vi "Multi_Run_Prog.vi"(0 "Command filename":path, 1 "Setup mode":T9(ring)) -> ()   [LabVIEW 2011]
uses:
  Anemometry Sub Vis/Globals/Trav_pos_global.vi
  Anemometry Sub Vis/Globals/Meas_global.vi
  ADAM Client/Sub VIs/ADAM Controls/Traverse_Level_State.ctl
  Anemometry Sub Vis/Gen Trav/Route mapping/Route_mapping_global.vi
  Anemometry Sub Vis/Globals/Preference_global.vi
  ADAM Client/Sub VIs/ADAM Controls/Client_Source_Status.ctl
  Anemometry Sub Vis/Controls/Multi_Run_Case.ctl
  Anemometry Sub Vis/Controls/User_Specific_mode.ctl
  ADAM Client/Sub VIs/ADAM Controls/Update_scan_value.ctl
  Anemometry Sub Vis/Controls/Multi_run_mode.ctl
  Anemometry Sub Vis/Gen Trav/Multi_Run_Status.ctl
  Anemometry Sub Vis/Globals/Extra_Commands_Global.vi
  Anemometry Sub Vis/Globals/LDA_meas_global_1.vi
  Anemometry Sub Vis/Globals/LDA_meas_global_2.vi
  ADAM Client/Sub VIs/ADAM Controls/Tunnel_speed_mode.ctl
  ADAM Client/Sub VIs/ADAM Controls/Remember_value_mode.ctl
  Anemometry Sub Vis/Controls/Overhead.ctl
  Anemometry Sub Vis/Controls/Post_Process.ctl
  Anemometry Sub Vis/Gen Trav/Spacing.ctl
  Anemometry Sub Vis/Gen Trav/Traverse_cluster.ctl
  Anemometry Sub Vis/Gen Trav/Trav_mode.ctl
  Anemometry Sub Vis/File/Setup_Filetype.ctl
  Anemometry Sub Vis/Controls/Tunnel_Coordinates.ctl
  Anemometry Sub Vis/Gen Trav/Route mapping/Route_Display_Mode.ctl
panel:
  out "Last Row Run":i32
  in  "Stop after Repeats":bool
  in  "Jump Bad Positions":bool
  in  "Work in Tunnel Coordinates?":T1
  out "Current Overhead Factor":dbl format="%.3f"
  out "Estimated Completion time":string
  out "Max Tunnel Speed":dbl format="%.2f"
  out "Pause message":string
  in  "Pause":bool
  out "Non Starter":bool
  out "No of Rows":i32
  out "Status":T2
  in  "Synchronization Start No":i32=1 min=1 max=100
  out "Multi Run Case":T3
  out "Simulate/Run":T4
  in  "Display Mode":T5=enum."Display View on Crash"
  in  "stop":bool
  out "Currently on Row":i32
  in  "Table":T6[](array[typedef]) {"Row Duration (mins)" format="%#.1f"; "Row No" min=0; "Trace Gas Concentration (%)" min=0.0 format="%#.2f"; "Emission Rate (l/min)" format="%#.2f"; "Tunnel Speed" format="%#.2f"; "Start X" format="%#.2f"; "Start Y" format="%#.2f"; "Start Z" format="%#.2f"; "End X" format="%#.2f"; "End Y" format="%#.2f"; "End Z" format="%#.2f"; "Averaging time (min)" min=0.0 format="%#.2f"}
  # "X           Y            Z"
  # "Start"
  # "End"
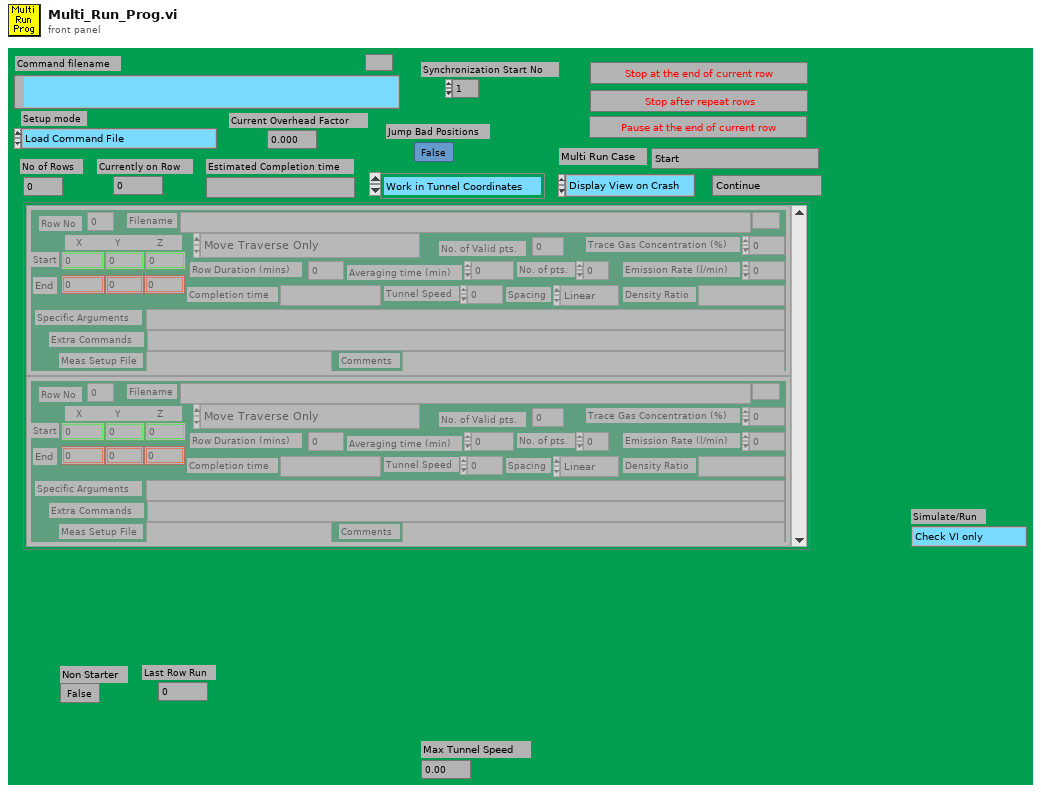
[diagram p1: front panel]
types:
  T1 = typedef "Tunnel_Coordinates.ctl" = enum16{"Work in Tunnel Coordinates", "Work in Model Coordinates"}
  T2 = typedef "Multi_Run_Status.ctl" = enum16{"Continue", "Jump to Next Point", "Jump to Next Row", "Jump To Fall Back", "Terminate Run"}
  T3 = typedef "Multi_Run_Case.ctl" = enum16{"Start", "Load Setup From File", "Has file been edited in Excel?", "Check Max Tunnel Speed", "Pre Check Row", "Check Rows", "Remove blank end rows", "Do results files already exist?", "FFID Bkgnd Measurements?", "First Save Setup file", "Setup Route checking", "Initialise Measurement Prog", "Input Current Position", "Experimental setup control", "Check source flowrates", "Setup for running mode", "Skip Blank Rows", "Which row to execute next", "Evaluate IF Statement", "Perform Measurement Setup", "Set Measurement Conditions", "Execute Row", "Calculate Row TIme", "Update time estimate", "Pause Multi Run Program", "Do Another Row?", "Find Next Fall Back Row", "Shut down source etc", "Email results to users", "Save run efficiency", "Remove Skipped Commands", "Show jumped positions", "Save Setup to File", "End"}
  T4 = typedef "User_Specific_mode.ctl" = enum16{"Check VI only", "Run VI"}
  T5 = typedef "Route_Display_Mode.ctl" = enum16{"Display View Always", "Display View on Crash"}
  T6 = typedef "Traverse_cluster.ctl" = cluster{"Start X":dbl, "Start Y":dbl, "Start Z":dbl, "End X":dbl, "End Y":dbl, "End Z":dbl, "No. of pts.":i32, "Spacing":T7, "Filename":path, "Tunnel Speed":dbl, "Averaging time (min)":dbl, "Extra Commands":string, "Specific Arguments":string, "Emission Rate (l/min)":dbl, "Trace Gas Concentration (%)":dbl, "Density Ratio":string, "Comments":string, "Row No":i32, "Row Type Selector":T8, "Completion time":string, "Row Duration (mins)":dbl, "No. of Valid pts.":i32, "Meas Setup File":string}
  T7 = typedef "Spacing.ctl" = enum16{"Linear", "Log", "Gauss", "Specified", "N/A"}
  T8 = typedef "Multi_run_mode.ctl" = enum16{"Move Traverse Only", "Set Tunnel Speed Only", "Set Source Only", "Set Measurement Conditions", "Single Measurement", "Vertical Profile", "Lateral Profile", "Longitudinal Profile", "Explore Volume", "Multi-Axis Profile", "Auto Calibrate", "Meas Fast FID Bkgnd", "Check Beam Power", "Scanning Valve Measurement", "Run VI Named:", "Set ADAM Ch", "Wait (minutes)", "Send Message", "Synchronize With:", "Fall Back to this Row", "Turn Off Row Repeating", "Blank Row"}
  T9 = enum16{"Load Command File", "Save Command File", "Check Multi Run Prog", "Check Multi Run Prog With Live Moves", "Run Multi Run Prog"}
  T10 = typedef "Post_Process.ctl" = enum16{"Take New Data", "Post Process Raw Data File"}
  T11 = typedef "Traverse_Level_State.ctl" = enum16{"Running", "Complete"}
  T12 = enum32{"existing file", "new file", "new or existing file", "existing dir", "new dir", "new or existing dir", "existing file (use LLBs)", "new file (use LLBs)", "new or existing file (use LLBs)", "new or existing file or directory (use LLBs)"}
  T13 = typedef "Tunnel_speed_mode.ctl" = enum16{"Set Speed", "Set Speed then wait", "Is tunnel speed allowable?"}
  T14 = enum16{"All Channel Names", "Valid Channel Names"}
  T15 = typedef "Overhead.ctl" = enum16{"Update total times", "Read Current Overhead", "Re Scale totals to 3 hrs", "Initialise totals to 3hr"}
  T16 = typedef "Remember_value_mode.ctl" = enum16{"Read only", "Read and Write"}
  T17 = typedef "Trav_mode.ctl" = enum16{"Move traverse", "Read traverse position", "Teach Position"}
  T18 = typedef "Client_Source_Status.ctl" = enum16{"Not Using", "Using", "Must Have"}
  T19 = typedef "Update_scan_value.ctl" = cluster{"Channel Name":string, "New Value":dbl}
  T20 = typedef "Setup_Filetype.ctl" = enum16{"Measurement Setups", "Calibration Setups", "General", "Results File Plotter Setups", "Speed Calib Tweaks"}
  T21 = typedef "Status_Cluster.ctl" = cluster{"Status":T2, "Error Type":string, "Error Description":string}
  T22 = typedef "BSA_info_Cluster.ctl" = cluster{"GPIB Address":string, "No of Check Bytes":i32, "Extra Info":string, "COLOUR":u32, "Wavelength (nm)":dbl}
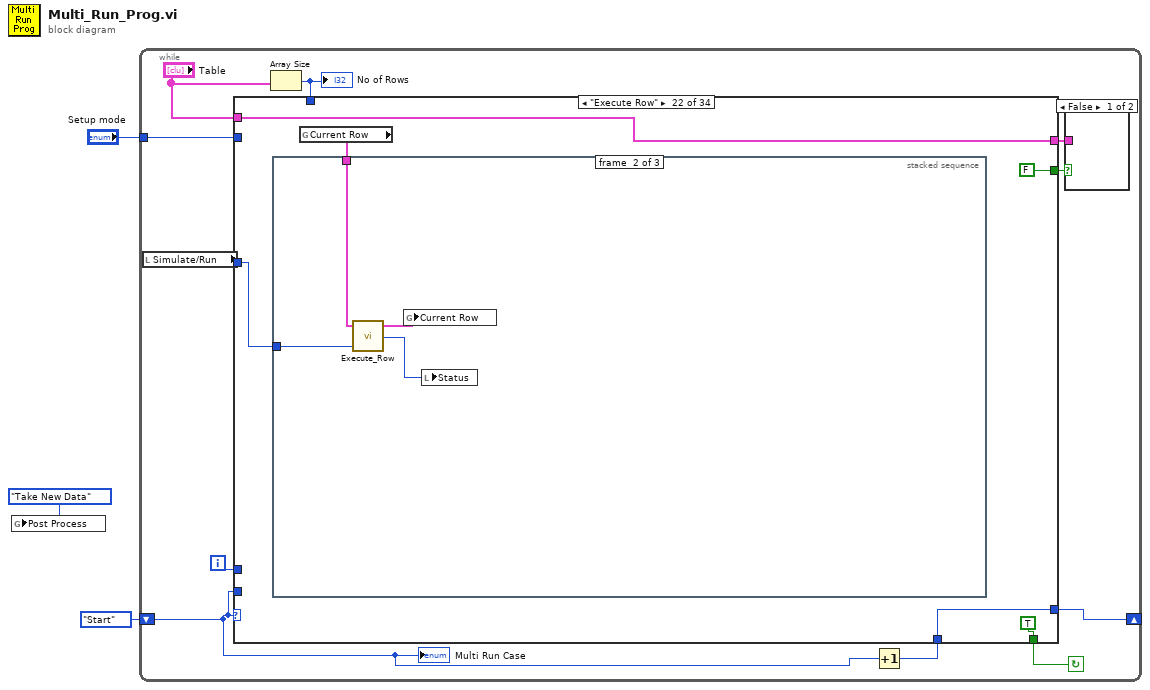
[diagram p0: block diagram]
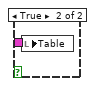
[diagram p2: hidden frame]
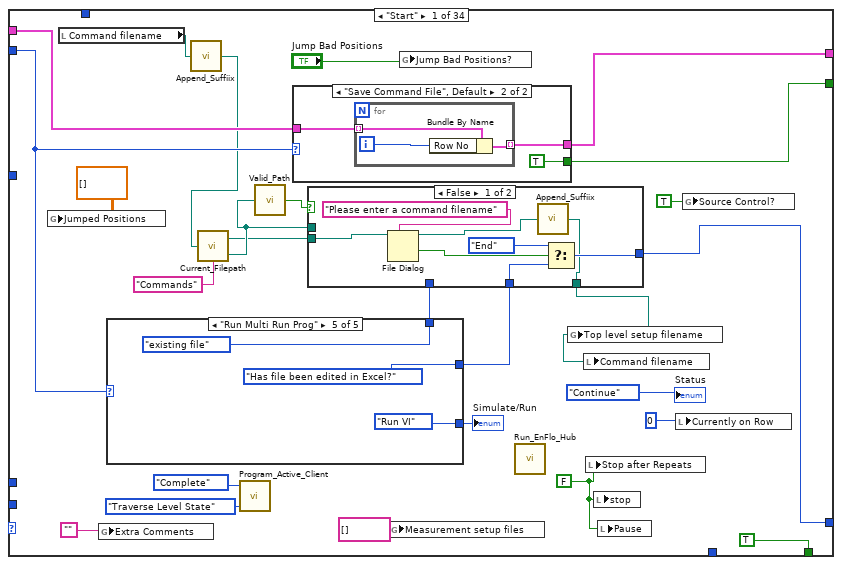
[diagram p3: hidden frame]
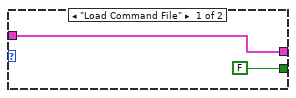
[diagram p4: hidden frame]
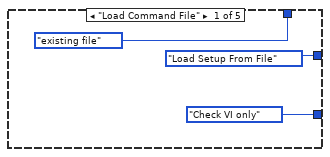
[diagram p6: hidden frame]
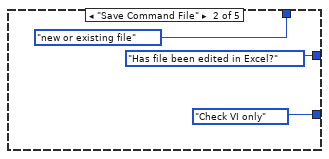
[diagram p7: hidden frame]
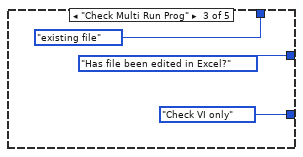
[diagram p8: hidden frame]
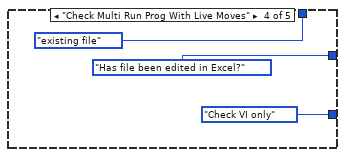
[diagram p9: hidden frame]
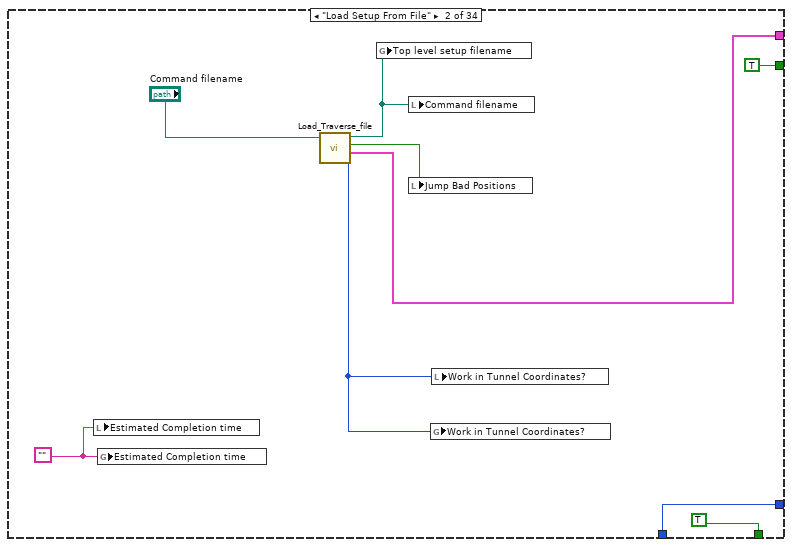
[diagram p10: hidden frame]
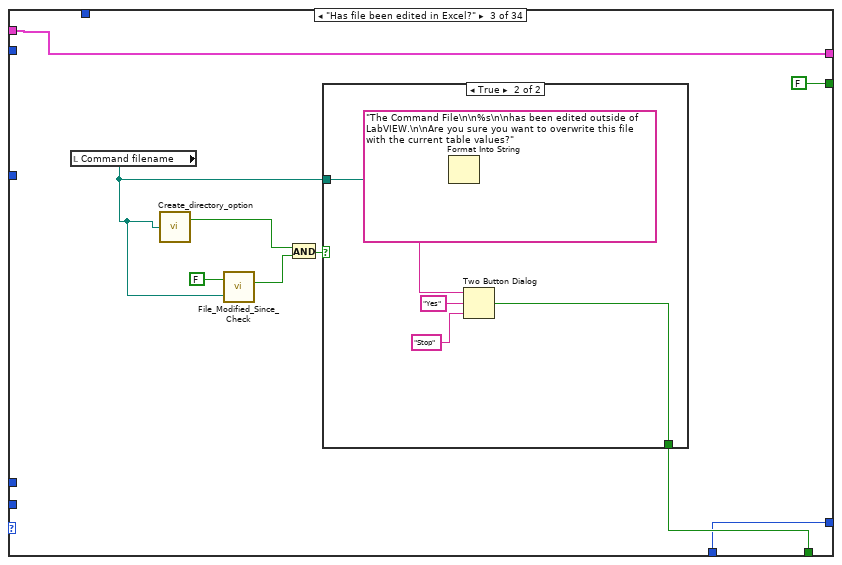
[diagram p11: hidden frame]
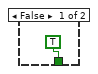
[diagram p12: hidden frame]
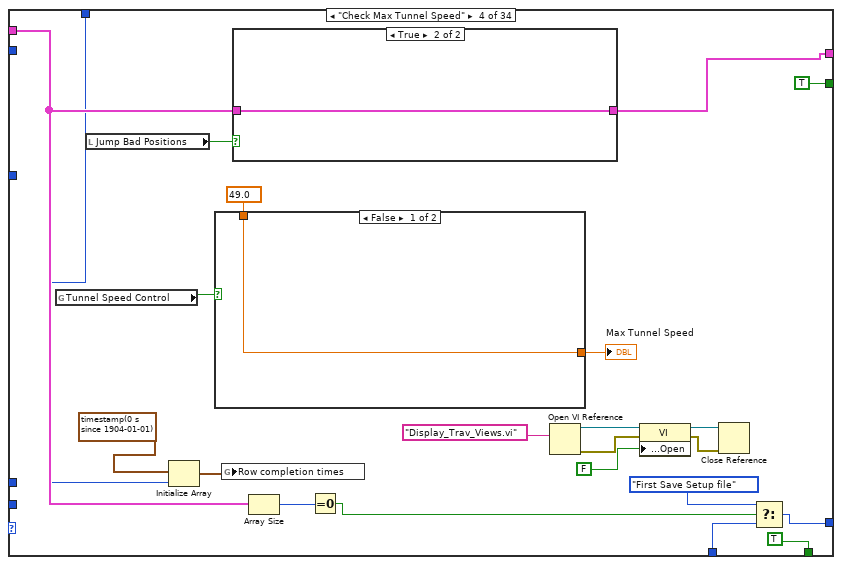
[diagram p13: hidden frame]
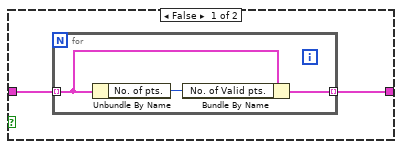
[diagram p14: hidden frame]
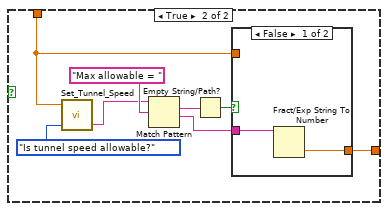
[diagram p15: hidden frame]
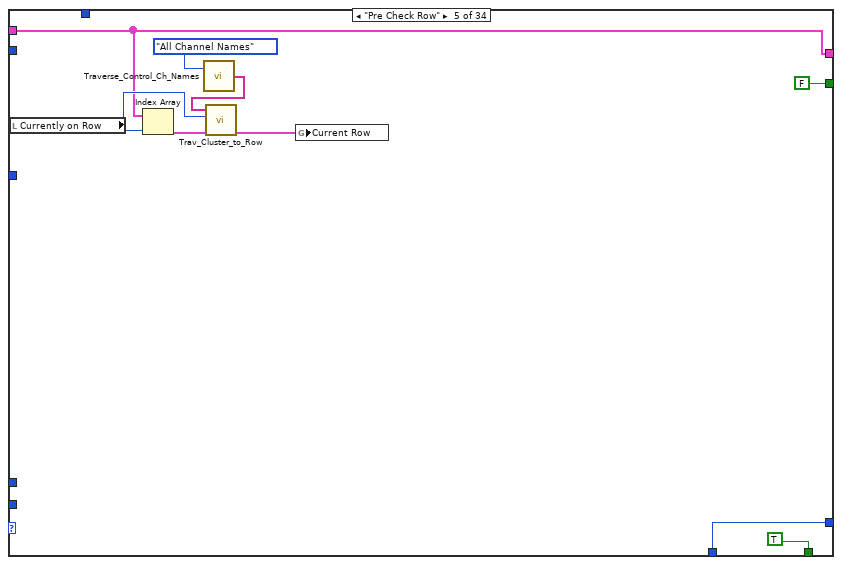
[diagram p17: hidden frame]
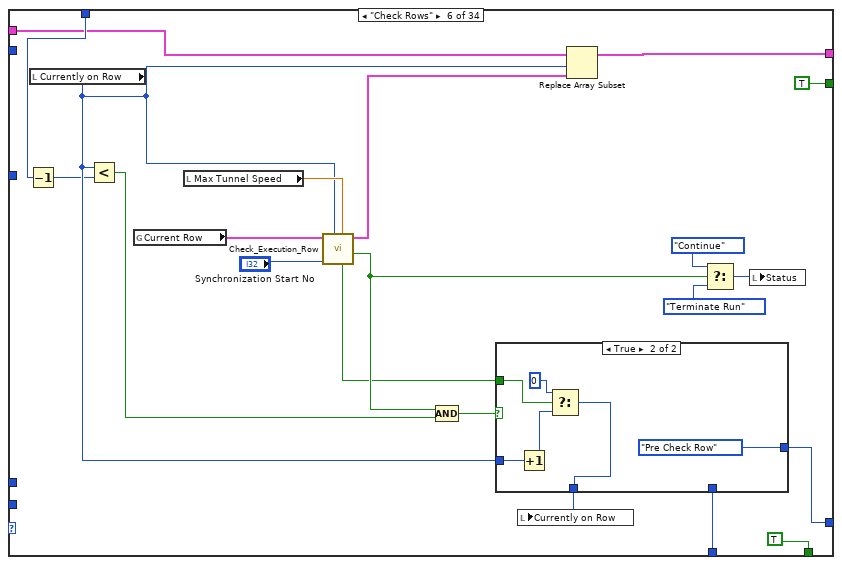
[diagram p18: hidden frame]
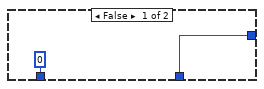
[diagram p19: hidden frame]
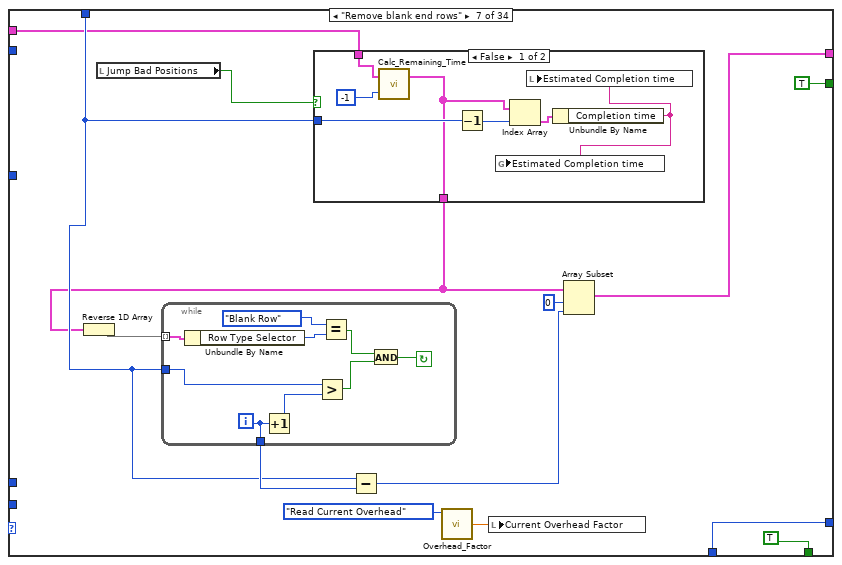
[diagram p20: hidden frame]
diagram:
  n1 = global write "Meas_global.vi" "Post Process"(Post_Process."Take New Data" ("Post Process")) -> ()
  n2 = while {
    shift-left: Multi_Run_Case."Start" ("Multi Run Case") -> [w10]
    shift-right: [w6] -> _
    tunnel: "Setup mode" -> [w13]
    i -> [w11]
    stop <- w14 continue-if-true
    n3 = local read "Simulate/Run"() -> (w7:T4)
    n4 = Array Size(array="Table") -> (size(s)=w5:i32)
    "No of Rows" <- w5
    n5 = Increment(x=w10) -> (x+1=w12:T3)
    n6 = case shown="\"Execute Row\"" w10 {
      tunnel: [TRUE TRUE w87 TRUE TRUE TRUE TRUE TRUE TRUE TRUE TRUE ("Continue?") TRUE ("Continue?") TRUE TRUE TRUE w508 TRUE ("Continue?") TRUE ("Continue?") TRUE TRUE ("Continue?") TRUE TRUE TRUE TRUE TRUE TRUE TRUE TRUE TRUE TRUE TRUE TRUE TRUE FALSE] -> w14
      tunnel: w13 -> [w26 _ _ _ _ _ _ _ _ w395 _ _ _ _ _ _ _ _ _ _ _ _ _ _ _ _ _ _ _ _ _ _ w1222 _]
      tunnel: "Table" -> [w39 _ w84 w114 w142 w154 w179 w210 w368 w397 w416 w444 w457 w485 w495 w511 w563 w607 w723 w774 w786 w877 w913 w945 w986 w1028 w1063 w1093 w1122 w1167 w1172 w1181 w1243 w1306]
      tunnel: w7 -> [_ _ _ _ _ _ _ w209 _ _ _ _ _ w489 w494 w510 _ w605 w720 w771 w784 w876 w911 w942 _ w1037 _ w1084 _ _ _ _ w1233 _]
      tunnel: w10 -> [_ _ _ _ _ _ _ _ _ _ _ _ _ _ _ _ _ _ _ _ _ _ _ _ _ _ _ _ _ _ _ _ _ _]
      tunnel: w12 -> [_ w80 w86 w112 w146 w156 w190 w214 w363 w394 w420 w441 w458 w484 w500 w513 w565 w603 w728 w775 w793 w874 w903 w947 w989 _ _ w1077 w1124 w1169 w1175 w1189 w1241 w1305]
      tunnel: w11 -> [_ _ _ _ _ _ _ _ _ _ _ _ _ _ _ _ _ _ _ _ _ _ _ _ w987 _ _ _ _ _ _ _ _ _]
      tunnel: [w37 w80 w86 w111 w146 w155 w190 w214 w363 w390 w420 w440 w458 w484 w497 w513 w565 w604 w727 w775 w794 w874 w903 w947 w990 w1038 w1060 w1088 w1124 w1169 w1175 w1189 w1241 w1305] -> w6
      tunnel: [w25 TRUE FALSE ("Rows Added ?") TRUE ("Rows Added ?") FALSE TRUE TRUE FALSE FALSE TRUE FALSE FALSE FALSE FALSE FALSE TRUE FALSE ("Rows Added ?") FALSE ("Rows Added ?") FALSE FALSE ("Rows Added ?") FALSE FALSE FALSE TRUE ("Rows Added ?") FALSE FALSE FALSE FALSE FALSE FALSE TRUE TRUE TRUE FALSE] -> w8
      tunnel: w5 -> [_ _ _ w106 _ w160 w181 _ _ _ _ _ _ _ _ _ w566 w606 _ _ _ _ _ w941 _ w1023 _ _ _ _ _ _ _ _]
      tunnel: [w38 w81 w84 w116 w142 w163 w185 w210 w368 w398 w416 w444 w457 w485 w495 w509 w563 w608 w723 w774 w786 w877 w913 w944 w986 w1028 w1063 w1093 w1122 w1167 w1171 w1181 w1242 w1306] -> w4
      frame "Start" {
        w23 = FALSE ("Measurment setup Found?")
        n7 = global write "Trav_pos_global.vi" "Jumped Positions"(dbl[][] [] ("Jumped Positions")) -> ()
        n8 = local read "Command filename"() -> (w29:path)
        n9 = global write "Meas_global.vi" "Extra Comments"("") -> ()
        n10 = case shown="\"Run Multi Run Prog\"" w26 {
          tunnel: [User_Specific_mode."Check VI only" ("Simulate/Run") User_Specific_mode."Check VI only" ("Simulate/Run") User_Specific_mode."Check VI only" ("Simulate/Run") User_Specific_mode."Check VI only" ("Simulate/Run") User_Specific_mode."Run VI" ("Simulate/Run")] -> w40
          tunnel: [Multi_Run_Case."Load Setup From File" ("Multi Run Case") Multi_Run_Case."Has file been edited in Excel?" ("Multi Run Case") Multi_Run_Case."Has file been edited in Excel?" ("Multi Run Case") Multi_Run_Case."Has file been edited in Excel?" ("Multi Run Case") Multi_Run_Case."Has file been edited in Excel?" ("Multi Run Case")] -> w36
          tunnel: [T12."existing file" ("select mode (2)") T12."new or existing file" ("select mode (2)") T12."existing file" ("select mode (2)") T12."existing file" ("select mode (2)") T12."existing file" ("select mode (2)")] -> w24
          frame "Load Command File" {
          }
          frame "Save Command File" {
          }
          frame "Check Multi Run Prog" {
          }
          frame "Check Multi Run Prog With Live Moves" {
          }
          frame "Run Multi Run Prog" {
          }
        }
        "Simulate/Run" <- w40
        n11 = call "Append_Suffiix.vi"("Results file"=w29) -> ("appended path"=w18:path)
        n12 = call "Current_Filepath.vi"("Filename in"=w18, "Data Type"="Commands") -> ("Filename Out"=w17:path, "Directory"=w16:path)
        n13 = call "Program_Active_Client.vi"("Mode"=enum16{"Program Active", "Traverse Level State"}."Traverse Level State", "Traverse level State"=Traverse_Level_State."Complete") -> ()  [unwired: 1 in, 3 out]
        n14 = call "Valid_Path.vi"("Filename"=w17) -> ("Valid Path?"=w27:bool)
        n15 = case shown="\"Save Command File\", Default" w26 {
          tunnel: w39 -> [w43 w46]
          tunnel: [w43 w45] -> w38
          tunnel: [FALSE TRUE] -> w25
          frame "Load Command File" {
          }
          frame "Save Command File", Default {
            n16 = for {
              tunnel: w46 -> [w49] mode=indexing
              tunnel: [w48] -> w45 mode=indexing
              i -> [w47]
              n17 = Bundle By Name(cluster=w49, "Row No"=w47) -> (w48:T6)
            }
          }
        }
        n18 = case shown="False" w27 {
          tunnel: [w55 w59] -> w37
          tunnel: w36 -> [w56 w59]
          tunnel: w17 -> [_ w58]
          tunnel: [w54 w58] -> w28
          tunnel: w24 -> [_ _]
          tunnel: w16 -> [w50 _]
          frame False {
            n19 = File Dialog(7:"Please enter a command filename" ("prompt"), 11:w50) -> (1:w52:bool, 3:w53:path)  [unwired: 1 in, 6 out]
            n20 = call "Append_Suffiix.vi"("Results file"=w53) -> ("appended path"=w54:path)
            n21 = Select(t=Multi_Run_Case."End" ("Multi Run Case"), s=w52, f=w56) -> (s? t:f=w55:T3)
          }
          frame True {
          }
        }
        n22 = global write "Trav_pos_global.vi" "Measurement setup files"(string[] [] ("Measurement setup files")) -> ()
        n23 = global write "Trav_pos_global.vi" "Jump Bad Positions?"("Jump Bad Positions") -> ()
        n24 = call "Run_EnFlo_Hub.vi"() -> ()  [unwired: 8 out]
        n25 = global write "Trav_pos_global.vi" "Top level setup filename"(w28) -> ()
        n26 = local write "Command filename"(w28) -> ()
        n27 = local write "Stop after Repeats"(w23) -> ()
        n28 = local write "stop"(w23) -> ()
        n29 = local write "Pause"(w23) -> ()
        n30 = local write "Currently on Row"(0 ("Currently on Row")) -> ()
        n31 = global write "Trav_pos_global.vi" "Source Control?"(TRUE ("Source Control?")) -> ()
        "Status" <- Multi_Run_Status."Continue" ("Status")
      }
      frame "Load Setup From File" {
        w76 = ""
        n32 = local write "Estimated Completion time"(w76) -> ()
        n33 = global write "Trav_pos_global.vi" "Estimated Completion time"(w76) -> ()
        n34 = call "Load_Traverse_file.vi"("Setup filename"="Command filename") -> ("Setup filename Out"=w78:path, "Jump Bad Positions"=w75:bool, "Table"=w81:T6[], "Work in Tunnel Coordinates?"=w77:T1)  [unwired: 2 out]
        n35 = global write "Trav_pos_global.vi" "Top level setup filename"(w78) -> ()
        n36 = local write "Command filename"(w78) -> ()
        n37 = local write "Jump Bad Positions"(w75) -> ()
        n38 = global write "Trav_pos_global.vi" "Work in Tunnel Coordinates?"(w77) -> ()
        n39 = local write "Work in Tunnel Coordinates?"(w77) -> ()
      }
      frame "Has file been edited in Excel?" {
        n40 = local read "Command filename"() -> (w88:path)
        n41 = call "Create_directory_option.vi"("Filename"=w88) -> ("Path is to existing File"=w91:bool)  [unwired: 1 out]
        n42 = call "File_Modified_Since_Check.vi"("Pathname"=w88, "Just Modified?"=FALSE) -> ("Modified?"=w90:bool)
        n43 = And(x=w91, y=w90) -> (x .and. y?=w92:bool)
        n44 = case shown="True" w92 {
          tunnel: w88 -> [_ w99]
          tunnel: [TRUE ("T button?") w94] -> w87
          frame False {
          }
          frame True {
            n45 = Format Into String(format string="The Command File\n\n%s\n\nhas been edited outside of LabVIEW.\n\nAre you sure you want to overwrite this file  with the current table values?" ("Format String"), w99) -> (resulting string=w97:string)  [unwired: 2 in, 1 out]
            n46 = Two Button Dialog(message=w97, 1:"Stop" ("F button name (\"Cancel\")"), 2:"Yes" ("T button name (\"OK\")")) -> (T button?=w94:bool)
          }
        }
      }
      frame "Check Max Tunnel Speed" {
        n47 = global read "Preference_global.vi" "Tunnel Speed Control"() -> (w117:bool)
        n48 = local read "Jump Bad Positions"() -> (w115:bool)
        n49 = Initialize Array(timestamp(0 s since 1904-01-01) ("seconds since 1Jan1904"), w106) -> (w107:timestamp[])
        n50 = case shown="False" w117 {
          tunnel: 49.0 ("Tunnel Velocity m/s") -> [w128 w129]
          tunnel: [w128 w131] -> w119
          frame False {
          }
          frame True {
            n51 = call "Set_Tunnel_Speed.vi"("Mode"=Tunnel_speed_mode."Is tunnel speed allowable?", "Tunnel Velocity m/s"=w129) -> ("Error String"=w134:string)  [unwired: 1 in, 2 out]
            n52 = Match Pattern(string=w134, regular expression="Max allowable = ") -> (match substring=w133:string, after substring=w130:string)  [unwired: 3 out]
            n53 = Empty String/Path?(string/path=w133) -> (empty?=w132:bool)
            n54 = case shown="False" w132 {
              tunnel: [w137 w139] -> w131
              tunnel: w129 -> [_ w139]
              tunnel: w130 -> [w138 _]
              frame False {
                n55 = Fract/Exp String To Number(string=w138) -> (number=w137:dbl)  [unwired: 4 out]
              }
              frame True {
              }
            }
          }
        }
        "Max Tunnel Speed" <- w119
        n56 = global write "Trav_pos_global.vi" "Row completion times"(w107) -> ()
        n57 = case shown="True" w115 {
          tunnel: w114 -> [w123 w127]
          tunnel: [w122 w127] -> w116
          frame False {
            n58 = for {
              tunnel: w123 -> [w125] mode=indexing
              tunnel: [w124] -> w122 mode=indexing
              n59 = Unbundle By Name(w125) -> ("No. of pts."=w126:i32)
              n60 = Bundle By Name(cluster=w125, "No. of Valid pts."=w126) -> (w124:T6)
            }
          }
          frame True {
          }
        }
        n61 = Array Size(array=w114) -> (size(s)=w113:i32)
        n62 = Equal To 0?(x=w113) -> (x = 0?=w110:bool)
        n63 = Open VI Reference(vi path="Display_Trav_Views.vi" ("VI path")) -> (vi reference=w105:refnum<vi>, error out=w104:errorcluster)  [unwired: 1 in, 4 out]
        n64 = property class="VI"(reference=w105, error in=w104, "Front Panel Window:Open"=FALSE) -> (reference out=w102:refnum<vi>, error out=w101:errorcluster)
        n65 = Close Reference(reference=w102, error in (no error)=w101) -> ()  [unwired: 1 out]
        n66 = Select(t=Multi_Run_Case."First Save Setup file" ("Multi Run Case"), s=w110, f=w112) -> (s? t:f=w111:T3)
      }
      frame "Pre Check Row" {
        n67 = local read "Currently on Row"() -> (w143:i32)
        n68 = Index Array(array=w142, index=w143) -> (element=w144:T6)
        n69 = call "Traverse_Control_Ch_Names.vi"("Mode"=T14."All Channel Names") -> ("Channel names"=w140:string[])  [unwired: 1 in]
        n70 = call "Trav_Cluster_to_Row.vi"("Traverse line in"=w144, "Row Number"=w143, "Channel names"=w140) -> ("Traverse line Out"=w145:T6)  [unwired: 4 out]
        n71 = global write "Trav_pos_global.vi" "Current Row"(w145) -> ()
      }
      frame "Check Rows" {
        n72 = Decrement(x=w160) -> (x-1=w150:i32)
        n73 = local read "Currently on Row"() -> (w151:i32)
        n74 = Less?(x=w151, y=w150) -> (x < y?=w159:bool)
        n75 = global read "Trav_pos_global.vi" "Current Row"() -> (w152:T6)
        n76 = local read "Max Tunnel Speed"() -> (w162:dbl)
        n77 = call "Check_Execution_Row.vi"("Execution Row"=w152, "Synchronization Start No"="Synchronization Start No", "Row Index"=w151, "Max Tunnel Speed"=w162) -> ("Editted Row"=w149:bool, "Execution Row Out"=w153:T6, "Continue?"=w161:bool)  [unwired: 1 in, 3 out]
        n78 = Compound Arithmetic op=AND(w161, w159) -> (w158:bool)
        n79 = case shown="True" w158 {
          tunnel: [0 w173] -> w157
          tunnel: w151 -> [_ w177]
          tunnel: w156 -> [w171 _]
          tunnel: [w171 Multi_Run_Case."Pre Check Row" ("Multi Run Case")] -> w155
          tunnel: w149 -> [_ w175]
          frame False {
          }
          frame True {
            n80 = Increment(x=w177) -> (x+1=w174:i32)
            n81 = Select(t=0, s=w175, f=w174) -> (s? t:f=w173:i32)
          }
        }
        n82 = local write "Currently on Row"(w157) -> ()
        n83 = Replace Array Subset(array=w154, new element=w153, index=w151) -> (w163:T6[])
        n84 = Select(t=Multi_Run_Status."Continue" ("Status"), s=w161, f=Multi_Run_Status."Terminate Run" ("Status")) -> (s? t:f=w167:T2)
        n85 = local write "Status"(w167) -> ()
      }
      frame "Remove blank end rows" {
        n86 = local read "Jump Bad Positions"() -> (w178:bool)
        n87 = case shown="False" w178 {
          tunnel: w181 -> [w196 _]
          tunnel: w179 -> [w195 w199]
          tunnel: [w193 w199] -> w180
          frame False {
            n88 = call "Calc_Remaining_Time.vi"("Currently on Row"=-1 ("Start Index"), "Table In"=w195) -> ("Table Out"=w193:T6[])  [unwired: 1 out]
            n89 = Decrement(x=w196) -> (x-1=w198:i32)
            n90 = Index Array(array=w193, index=w198) -> (element=w197:T6)
            n91 = Unbundle By Name(w197) -> ("Completion time"=w192:string)
            n92 = global write "Trav_pos_global.vi" "Estimated Completion time"(w192) -> ()
            n93 = local write "Estimated Completion time"(w192) -> ()
          }
          frame True {
          }
        }
        n94 = Reverse 1D Array(array=w180) -> (reversed array=w189:T6[])
        n95 = while {
          tunnel: [w200] -> w187
          tunnel: w181 -> [w204]
          tunnel: w189 -> [w208] mode=indexing
          i -> [w200]
          stop <- w201 continue-if-true
          n96 = Unbundle By Name(w208) -> ("Row Type Selector"=w206:T8)
          n97 = Increment(x=w200) -> (x+1=w205:i32)
          n98 = Greater?(x=w204, y=w205) -> (0:w203:bool)
          n99 = Equal?(x=Multi_run_mode."Blank Row" ("Row Type Selector"), y=w206) -> (x = y?=w202:bool)
          n100 = And(x=w202, y=w203) -> (x .and. y?=w201:bool)
        }
        n101 = Subtract(x=w181, y=w187) -> (x-y=w186:i32)
        n102 = call "Overhead_Factor.vi"("Mode"=Overhead."Read Current Overhead") -> ("Current Overhead Factor"=w182:dbl)  [unwired: 3 in]
        n103 = local write "Current Overhead Factor"(w182) -> ()
        n104 = Array Subset(array=w180, index=0 ("Array Index"), length=w186) -> (w185:T6[])
      }
      frame "Do results files already exist?" {
        n105 = for {
          tunnel: w210 -> [w226] mode=indexing
          tunnel: [w224] -> w216 mode=indexing
          shift-right: [w220] -> _
          shift-left: path[] [] -> [w221]
          tunnel: w209 -> [w218]
          n106 = Unbundle By Name(w226) -> ("Specific Arguments"=w217:string, "Emission Rate (l/min)"=w225:dbl, "Row Type Selector"=w223:T8, "Filename"=w222:path)
          n107 = while {
            shift-left: w221 -> [w234]
            shift-right: [w233] -> w220
            tunnel: w222 -> [w235]
            tunnel: w223 -> [w239]
            shift-left: 0 -> [w240]
            shift-right: [w236] -> _
            tunnel: w218 -> [w230]
            shift-right: [w229] -> _
            shift-left: _ -> [w228]
            tunnel: w217 -> [w227]
            stop <- w238 continue-if-true
            n108 = Increment(x=w240) -> (x+1=w237:i32)
            n109 = case shown="0, Default" w240 {
              tunnel: w239 -> [w249 _ _ _ _ _ _ _ _ _ _ _]
              tunnel: [w244 w269 w274 w281 w286 TRUE ("exists?") TRUE ("exists?") FALSE ("exists?") FALSE ("exists?") TRUE ("true") w343 w356] -> w238
              tunnel: w237 -> [w251 w272 w277 w280 w287 w292 w303 w314 w325 w329 w341 _]
              tunnel: [w251 w272 w277 w280 w287 w290 w302 w314 w325 w330 w341 w355] -> w236
              tunnel: [w250 w271 w276 w279 w284 w300 w311 w316 w318 w327 w345 w361] -> w233
              tunnel: w234 -> [w250 w271 w276 w279 w285 w300 w311 w316 w318 w327 w345 w361]
              tunnel: w235 -> [w243 _ _ _ _ _ _ _ _ _ _ _]
              tunnel: 7 -> [_ _ _ _ _ _ _ _ _ w328 _ w355]
              tunnel: 9 -> [_ _ _ _ _ w291 _ _ _ _ _ _]
              tunnel: w230 -> [_ _ _ _ _ _ _ _ _ _ w344 _]
              tunnel: [w242 w268 w273 w278 w283 w288 w301 w312 w317 w326 w342 w354] -> w229
              tunnel: w228 -> [_ w268 w273 w278 w283 w288 w301 w312 w317 w326 w342 w354]
              tunnel: w227 -> [w241 _ _ _ _ _ _ _ _ _ _ _]
              frame 0, Default {
                n110 = case shown="\"Run VI Named:\"" w249 {
                  tunnel: [TRUE w259 FALSE FALSE] -> w246
                  tunnel: w243 -> [w252 w258 w264 w266]
                  tunnel: w241 -> [_ w256 _ _]
                  tunnel: [w252 w258 w264 w266] -> w242
                  frame "Move Traverse Only", Default {
                  }
                  frame "Run VI Named:" {
                    n111 = Match Pattern(string=w256, regular expression=";") -> (before substring=w255:string)  [unwired: 4 out]
                    n112 = call <vilib>:"Trim Whitespace.vi"("string"=w255) -> ("trimmed string"=w254:string)  [unwired: 1 in]
                    n113 = Equal?(x=w254, y="Pressure_Tapped_Cube.vi") -> (x = y?=w260:bool)
                    n114 = Equal?(x=w254, y="Take_Data_on_the_Move.vi") -> (x = y?=w261:bool)
                    n115 = Or(x=w260, y=w261) -> (x .or. y?=w259:bool)
                  }
                  frame "Auto Calibrate" {
                  }
                  frame "Send Message" {
                  }
                }
                n116 = local read "Status"() -> (w247:T2)
                n117 = Not Equal?(x=Multi_Run_Status."Terminate Run" ("Status"), y=w247) -> (x != y?=w245:bool)
                n118 = And(x=w246, y=w245) -> (x .and. y?=w244:bool)
              }
              frame 1 {
                n119 = Not Equal?(x=path "", y=w268) -> (x != y?=w269:bool)
              }
              frame 2 {
                n120 = Not Equal?(x=w273, y=path "") -> (x != y?=w274:bool)
              }
              frame 3 {
                n121 = Search 1D Array(1D array=w279, element=w278) -> (index of element=w282:i32)  [unwired: 1 out]
                n122 = Less Than 0?(x=w282) -> (x < 0?=w281:bool)
              }
              frame 4 {
                n123 = Build Array (concatenate)(w285, w283) -> (w284:path[])
                n124 = call "Does_file_exist_(simple).vi"("Pathname"=w283) -> ("exists?"=w286:bool)
              }
              frame 5 {
                n125 = Path To String(path=w288) -> (string=w299:string)
                n126 = global read "Meas_global.vi" "Start Time of experiment"() -> (w294:dbl)
                n127 = Concatenate Strings(w299, "Append" ("Substring")) -> (w297:string)
                n128 = call "Remember_value.vi"("Mode"=Remember_value_mode."Read only", "Ch name"=w297) -> ("Output Value"=w295:dbl)  [unwired: 1 in]
                n129 = Not Equal?(x=w294, y=w295) -> (x != y?=w293:bool)
                n130 = Select(t=w292, s=w293, f=w291) -> (s? t:f=w290:i32)
              }
              frame 6 {
                n131 = Increment(x=w303) -> (x+1=w304:i32)
                n132 = Format Into String(format string="The results filename \"%s\" already exists.\nDo you wish to append to this file during the run?" ("Format String"), w301) -> (resulting string=w308:string)  [unwired: 2 in, 1 out]
                n133 = Two Button Dialog(message=w308, 1:"Abort Run" ("F button name (\"Cancel\")"), 2:"Append" ("T button name (\"OK\")")) -> (T button?=w305:bool)
                n134 = Select(t=w304, s=w305, f=w303) -> (s? t:f=w302:i32)
              }
              frame 7 {
                n135 = local write "Status"(Multi_Run_Status."Terminate Run" ("Status")) -> ()
              }
              frame 8 {
                n136 = Path To String(path=w317) -> (string=w324:string)
                n137 = Concatenate Strings(w324, "Append" ("Substring")) -> (w322:string)
                n138 = global read "Meas_global.vi" "Start Time of experiment"() -> (w319:dbl)
                n139 = call "Remember_value.vi"("Mode"=Remember_value_mode."Read and Write", "Input Value"=w319, "Ch name"=w322) -> ()  [unwired: 1 out]
              }
              frame 9 {
                n140 = call "Read_File_Simple.vi"("Filename"=w326) -> ("string"=w333:string)  [unwired: 2 in, 7 out]
                n141 = call "Is_it_a_Results_File.vi"("character string"=w333) -> ("Results File?"=w332:bool)  [unwired: 2 out]
                n142 = case shown="True" w332 {
                  tunnel: w326 -> [w336 _]
                  tunnel: [w334 w340] -> w330
                  tunnel: w329 -> [_ w340]
                  tunnel: w328 -> [w334 _]
                  frame False {
                    n143 = Path To String(path=w336) -> (string=w338:string)
                    n144 = Format Into String(format string="The File %s is not in the correct Results file format.\nCheck that it is tab delimited rather than excel format, or choose another file." ("Format String"), w338) -> (resulting string=w335:string)  [unwired: 2 in, 1 out]
                    n145 = One Button Dialog(message=w335, button name ("OK")="Stop") -> ()  [unwired: 1 out]
                  }
                  frame True {
                  }
                }
              }
              frame 10 {
                n146 = case shown="\"Check VI only\", Default" w344 {
                  tunnel: w342 -> [_ w353]
                  tunnel: [FALSE ("exists?") w347] -> w343
                  frame "Check VI only", Default {
                  }
                  frame "Run VI" {
                    n147 = call "Open_File_for_write.vi"("append to file? (new file:F)"=TRUE, "file path"=w353) -> ("error out"=w351:errorcluster, "refnum"=w352:refnum<file>)  [unwired: 1 in, 7 out]
                    n148 = Unbundle By Name(w351) -> ("code"=w350:i32)
                    n149 = Close File(refnum=w352, error in=w351) -> ()  [unwired: 2 out]
                    n150 = Equal?(x=10 ("code"), y=w350) -> (x = y?=w347:bool)
                  }
                }
              }
              frame 11 {
                n151 = Path To String(path=w354) -> (string=w359:string)
                n152 = Format Into String(format string="The File %s is already open in another application." ("Format String"), w359) -> (resulting string=w358:string)  [unwired: 2 in, 1 out]
                n153 = One Button Dialog(message=w358, button name ("OK")="Stop") -> (true=w356:bool)
              }
            }
          }
          n154 = Greater Than 0?(x=w225) -> (x > 0?=w224:bool)
        }
        n155 = Or Array Elements(Boolean array=w216) -> (logical OR=w212:bool)
        n156 = global write "Trav_pos_global.vi" "Source Control?"(w212) -> ()
      }
      frame "FFID Bkgnd Measurements?" {
        n157 = for {
          tunnel: w368 -> [w384] mode=indexing
          tunnel: [w372] -> w367 mode=indexing
          tunnel: [w373] -> w366 mode=indexing
          n158 = Unbundle By Name(w384) -> ("Row Type Selector"=w378:T8, "Specific Arguments"=w380:string)
          n159 = call "Get_array_values_fr_String.vi"("String Value"=w380) -> ("String array"=w381:string[])  [unwired: 1 out]
          n160 = Index Array(array=w381, index=0 ("Index")) -> (element=w377:string)
          n161 = Equal?(x=Multi_run_mode."Auto Calibrate" ("Row Type Selector"), y=w378) -> (x = y?=w374:bool)
          n162 = Equal?(x=w377, y="Concentration") -> (x = y?=w375:bool)
          n163 = Equal?(x=Multi_run_mode."Meas Fast FID Bkgnd" ("Row Type Selector"), y=w378) -> (x = y?=w372:bool)
          n164 = And(x=w374, y=w375) -> (x .and. y?=w373:bool)
        }
        n165 = Or Array Elements(Boolean array=w367) -> (logical OR=w364:bool)
        n166 = Or Array Elements(Boolean array=w366) -> (logical OR=w365:bool)
        n167 = Compound Arithmetic op=AND(invert w364, w365) -> (w362:bool)
        n168 = case shown="True" w362 {
          frame False {
          }
          frame True {
            n169 = One Button Dialog(message="This run automatically calibrates the Fast FID but does not have a Meas Fast FID Bkgnd row" ("format string")) -> ()  [unwired: 2 out]
          }
        }
      }
      frame "First Save Setup file" {
        w385 = -1 ("Currently on Row")
        n170 = case shown="\"Check Multi Run Prog\"" w395 {
          tunnel: [w402 w404 w406 Multi_Run_Case."End" ("Multi Run Case") Multi_Run_Case."End" ("Multi Run Case")] -> w389
          tunnel: w394 -> [w402 w404 w406 _ _]
          tunnel: [w403 w405 w407 w408 w410] -> w388
          frame "Run Multi Run Prog" {
            w403 = FALSE  # Live Traverse Preview?
          }
          frame "Check Multi Run Prog With Live Moves" {
            w405 = TRUE  # Live Traverse Preview?
          }
          frame "Check Multi Run Prog" {
            w407 = FALSE  # Live Traverse Preview?
          }
          frame "Load Command File" {
            w408 = FALSE  # Live Traverse Preview?
          }
          frame "Save Command File" {
            w410 = FALSE  # Live Traverse Preview?
          }
        }
        n171 = local read "Command filename"() -> (w396:path)
        n172 = global write "Trav_pos_global.vi" "Work in Tunnel Coordinates?"("Work in Tunnel Coordinates?") -> ()
        n173 = local write "Currently on Row"(w385) -> ()
        n174 = local write "Last Row Run"(w385) -> ()
        n175 = local read "Jump Bad Positions"() -> (w386:bool)
        n176 = call "Save_Trav_setup.vi"("Work in Tunnel Coordinates?"="Work in Tunnel Coordinates?", "Trav Table"=w397, "Jump Bad Positions"=w386, "Setup filename"=w396) -> ("Trav Table Out"=w398:T6[])  [unwired: 1 out]
        n177 = global write "Meas_global.vi" "Extra Comments"("") -> ()
        n178 = global write "Trav_pos_global.vi" "Live Traverse Preview?"(w388) -> ()
        n179 = local read "Status"() -> (w391:T2)
        n180 = case shown="\"Continue\"" w391 {
          tunnel: [w400 Multi_Run_Case."End" ("Multi Run Case")] -> w390
          tunnel: w389 -> [w400 _]
          frame "Continue" {
          }
          frame "Jump to Next Point", Default {
          }
        }
      }
      frame "Setup Route checking" {
        n181 = for {
          tunnel: w416 -> [w434] mode=indexing
          shift-right: [w425] -> w414
          shift-left: string[] [] -> [w426]
          n182 = Unbundle By Name(w434) -> ("Extra Commands"=w427:string, "Start X"=w431:dbl, "Start Y"=w430:dbl, "Start Z"=w429:dbl)
          n183 = Build Array(w431, w430, w429) -> (w432:dbl[])
          n184 = Not A Number/Path/Refnum?(number/path/refnum=w432) -> (NaN/Path/Refnum?=w433:bool[])
          n185 = Or Array Elements(Boolean array=w433) -> (logical OR=w428:bool)
          n186 = case shown="False" w428 {
            tunnel: w427 -> [w438 _]
            tunnel: w426 -> [w437 w439]
            tunnel: [w436 w439] -> w425
            frame False {
              n187 = call "Which_Trav_Setup.vi"("Extra Command String"=w438) -> ("Traverse Setup"=w435:string)
              n188 = Build Array (concatenate)(w437, w435) -> (w436:string[])
            }
            frame True {
            }
          }
        }
        n189 = call "Save_ADAM_Table_Locally.vi"() -> ()  [unwired: 12 in]
        n190 = global write "Route_mapping_global.vi" "Display Mode"("Display Mode") -> ()
        n191 = global read "Trav_pos_global.vi" "Work in Tunnel Coordinates?"() -> (w412:T1)
        n192 = call "Analyse_string_array.vi"("String array"=w414) -> ("Unique strings"=w413:string[])  [unwired: 2 out]
        n193 = for {
          tunnel: w413 -> [w424] mode=indexing
          tunnel: w412 -> [w421]
          n194 = call "3D_Traverse_move.vi"("Mode"=Trav_mode."Read traverse position", "Work in Tunnel Coordinates"=w421, "Simulate/Run"=User_Specific_mode."Run VI", "Traverse name"=w424) -> ()  [unwired: 5 in, 7 out]
        }
      }
      frame "Initialise Measurement Prog" {
        n195 = Array Size(array=w444) -> (size(s)=w445:i32)
        n196 = Decrement(x=w445) -> (x-1=w446:i32)
        n197 = while {
          tunnel: [w450] -> w442
          tunnel: User_Specific_mode."Check VI only" ("Simulate/Run") -> [w451]
          tunnel: w446 -> [w454]
          tunnel: w444 -> [w456] mode=indexing
          i -> [w455]
          stop <- w452 continue-if-true
          n198 = call "Perform_Meas_Setup.vi"("Simulate/Run"=w451, "Traverse line"=w456) -> ("Continue?"=w450:bool)  [unwired: 1 out]
          n199 = Less?(x=w455, y=w454) -> (x < y?=w453:bool)
          n200 = Compound Arithmetic op=AND(w450, w453) -> (w452:bool)
        }
        n201 = Select(t=w441, s=w442, f=Multi_Run_Case."End" ("Multi Run Case")) -> (s? t:f=w440:T3)
      }
      frame "Input Current Position" {
        n202 = disable-structure shown="Disabled" {
          disable-tunnel: w457 -> [w465 _]
          frame Disabled {
            n203 = global read "Trav_pos_global.vi" "Default Traverse Setup"() -> (w463:string)
            n204 = Build Array(w463) -> (w462:string[])
            n205 = global read "Extra_Commands_Global.vi" "!Traverse Setup"() -> (w464:string)
            n206 = for {
              tunnel: w465 -> [w478] mode=indexing
              tunnel: w464 -> [w476]
              shift-right: [w474] -> w461
              shift-left: w462 -> [w475]
              n207 = Unbundle By Name(w478) -> ("Extra Commands"=w477:string)
              n208 = call "Extra_Commands.vi"("String to Search"=w477, "Command"=w476) -> ("String Value"=w473:string, "Command Found"=w471:bool)  [unwired: 1 in, 3 out]
              n209 = Search 1D Array(1D array=w475, element=w473) -> (index of element=w470:i32)  [unwired: 1 out]
              n210 = Less Than 0?(x=w470) -> (x < 0?=w469:bool)
              n211 = And(x=w471, y=w469) -> (x .and. y?=w472:bool)
              n212 = case shown="True" w472 {
                tunnel: w475 -> [w479 w482]
                tunnel: [w479 w481] -> w474
                tunnel: w473 -> [_ w480]
                frame False {
                }
                frame True {
                  n213 = Build Array (concatenate)(w482, w480) -> (w481:string[])
                }
              }
            }
            n214 = for {
              tunnel: w461 -> [w467] mode=indexing
              n215 = call "Read_Traverse_Pos_File.vi"("Traverse Name"=w467) -> ("Tunnel Coordinates"=w466:dbl[])
              n216 = call "Read-Write_Check_Pos.vi"("Position input"=w466, "Mode"=enum16{"Read", "Write"}."Write", "Traverse Name"=w467) -> ()  [unwired: 1 out]
            }
          }
          frame Enabled {
          }
        }
      }
      frame "Experimental setup control" {
        n217 = global read "Trav_pos_global.vi" "Source Control?"() -> (w486:bool)
        n218 = Equal?(x=w489, y=User_Specific_mode."Run VI" ("Simulate/Run")) -> (x = y?=w488:bool)
        n219 = Or(x=w486, y=w488) -> (x .or. y?=w487:bool)
        n220 = case shown="True" w487 {
          tunnel: w486 -> [_ w493]
          frame False {
          }
          frame True {
            n221 = call "Exp_Setup_Control_remote.vi"("Dispersion?"=w493) -> ()  [unwired: 3 out]
          }
        }
        n222 = global write "Trav_pos_global.vi" "FFID Background"(T6 {"Start X"=nan, "Start Y"=nan, "Start Z"=nan, "End X"=nan, "End Y"=nan, "End Z"=nan, "No. of pts."=0, "Spacing"=enum."Linear", "Filename"=path "", "Tunnel Speed"=nan, "Averaging time (min)"=nan, "Extra Commands"="", "Specific Arguments"="", "Emission Rate (l/min)"=nan, "Trace Gas Concentration (%)"=nan, "Density Ratio"="", "Comments"="", "Row No"=0, "Row Type Selector"=enum."Blank Row", "Completion time"="", "Row Duration (mins)"=nan, "No. of Valid pts."=0, "Meas Setup File"=""} ("FFID Background")) -> ()
      }
      frame "Check source flowrates" {
        n223 = case shown="\"Run VI\"" w494 {
          tunnel: w495 -> [_ w504]
          frame "Check VI only", Default {
            n224 = Get Date/Time In Seconds() -> (seconds since 1Jan1904=w503:timestamp)
            n225 = global write "Trav_pos_global.vi" "Simulation Time"(w503) -> ()
          }
          frame "Run VI" {
            n226 = for {
              tunnel: w504 -> [w505] mode=indexing
              n227 = call "Set_Source.vi"("Source Status"=Client_Source_Status."Using", "Traverse line"=w505, "Simulate/Run"=User_Specific_mode."Check VI only") -> ()  [unwired: 1 in, 6 out]
            }
          }
        }
        n228 = Equal?(x=w494, y=User_Specific_mode."Run VI" ("Simulate/Run")) -> (x = y?=w498:bool)
        n229 = Increment(x=w500) -> (x+1=w496:T3)
        n230 = Select(t=w500, s=w498, f=w496) -> (s? t:f=w497:T3)
      }
      frame "Setup for running mode" {
        n231 = stacked-sequence {
          seq-local: [_ _ _ _ w541 _] -> [_ _ _ _ _ w559]
          tunnel: w511 -> [w516 _ _ w540 _ _]
          tunnel: w510 -> [_ _ w535 _ _ _]
          tunnel: [_ _ _ w538 _ _] -> w509
          tunnel: [_ _ _ _ w541 _] -> w508
          frame #0 {
            n232 = for {
              tunnel: w516 -> [w520] mode=indexing
              tunnel: [w517] -> w515 mode=indexing
              n233 = Unbundle By Name(w520) -> ("Row Type Selector"=w519:T8)
              n234 = Equal?(x=Multi_run_mode."Synchronize With:" ("Row Type Selector"), y=w519) -> (x = y?=w517:bool)
            }
            n235 = call "Setup_Environment.vi"() -> ()  [unwired: 1 in, 1 out]
            n236 = Or Array Elements(Boolean array=w515) -> (logical OR=w514:bool)
            n237 = case shown="True" w514 {
              frame False {
              }
              frame True {
                n238 = call "Declare_Sync_Client.vi"() -> ()  [unwired: 6 out]
              }
            }
          }
          frame #1 {
            n239 = Open VI Reference(vi path="Display_Trav_Views.vi" ("VI path")) -> (vi reference=w526:refnum<vi>, error out=w525:errorcluster)  [unwired: 1 in, 4 out]
            n240 = global write "Meas_global.vi" "Post Process"(Post_Process."Take New Data" ("Post Process")) -> ()
            n241 = property class="VI"(reference=w526, error in=w525, "Front Panel Window:Open"=FALSE) -> (reference out=w523:refnum<vi>, error out=w522:errorcluster)
            n242 = Close Reference(reference=w523, error in (no error)=w522) -> ()  [unwired: 1 out]
          }
          frame #2 {
            w530 = TRUE  # Start of Multi Run Prog
            w536 = TRUE
            n243 = Get Date/Time In Seconds() -> (seconds since 1Jan1904=w529:timestamp)
            n244 = To Double Precision Float(number=w529) -> (double precision float=w528:dbl)
            n245 = global write "Preference_global.vi" "Unblock Email"(w536) -> ()
            n246 = global write "Preference_global.vi" "Unblock SMS"(w536) -> ()
            n247 = global write "Meas_global.vi" "Start Time of experiment"(w528) -> ()
            n248 = local read "Command filename"() -> (w534:path)
            n249 = Path To String(path=w534) -> (string=w532:string)
            n250 = Concatenate Strings("Commencing a new multi run Prog having the setup filename of :" ("Message"), w532) -> (w531:string)
            n251 = call "Log_Current_row_to_Execute.vi"("Simulate/Run"=w535, "Message"=w531, "Start of Multi Run Prog"=w530) -> ()  [unwired: 2 in, 5 out]
          }
          frame #3 {
            n252 = call "Calc_Remaining_Time.vi"("Currently on Row"=-1, "Table In"=w540) -> ("Estimated Completion time"=w537:string, "Table Out"=w538:T6[])
            n253 = local write "Estimated Completion time"(w537) -> ()
            n254 = global write "Trav_pos_global.vi" "Estimated Completion time"(w537) -> ()
          }
          frame #4 {
            n255 = global read "Trav_pos_global.vi" "Source Control?"() -> (w542:bool)
            n256 = case shown="True" w542 {
              tunnel: [TRUE ("T button?") w547] -> w541
              frame False {
              }
              frame True {
                w548 = "EnFlo_Tunnel:Gas Solenoid:Status"
                n257 = Build Array(w548) -> (w551:string[])
                n258 = call "Get_Current_Scan_client.vi"("ADAM Ch Names"=w551) -> ("Numerical Values"=w550:dbl[])  [unwired: 3 out]
                n259 = Index Array(array=w550, index=0) -> (element=w546:dbl)
                n260 = Greater?(x=w546, y=0.5) -> (0:w544:bool)
                n261 = case shown="False" w544 {
                  tunnel: w548 -> [w557 _]
                  tunnel: [w552 TRUE ("T button?")] -> w547
                  frame False {
                    n262 = Format Into String(format string="The \"%s\" ADAM channel is showing that the blue gas button is not on.", w557) -> (resulting string=w555:string)  [unwired: 2 in, 1 out]
                    n263 = Two Button Dialog(message=w555, 1:"Stop" ("F button name (\"Cancel\")"), 2:"Continue" ("T button name (\"OK\")")) -> (T button?=w552:bool)
                  }
                  frame True {
                  }
                }
              }
            }
          }
          frame #5 {
            n264 = case shown="True" w559 {
              frame False {
              }
              frame True {
                n265 = call "Program_Active_Client.vi"("Mode"=enum16{"Program Active", "Traverse Level State"}."Traverse Level State", "Traverse level State"=Traverse_Level_State."Running") -> ()  [unwired: 1 in, 3 out]
              }
            }
          }
        }
      }
      frame "Skip Blank Rows" {
        n266 = stacked-sequence {
          tunnel: w566 -> [w569 w588]
          tunnel: w563 -> [w567 w584]
          frame #0 {
            n267 = Decrement(x=w569) -> (x-1=w568:i32)
            n268 = while {
              tunnel: w567 -> [w579]
              tunnel: w568 -> [w573]
              stop <- w570 continue-if-true
              n269 = local read "Currently on Row"() -> (w575:i32)
              n270 = Increment(x=w575) -> (x+1=w574:i32)
              n271 = Less?(x=w574, y=w573) -> (x < y?=w572:bool)
              n272 = Index Array(array=w579, index=w574) -> (element=w578:T6)
              n273 = Unbundle By Name(w578) -> ("Row Type Selector"=w577:T8)
              n274 = Equal?(x=Multi_run_mode."Blank Row" ("Row Type Selector"), y=w577) -> (x = y?=w571:bool)
              n275 = case shown="True" w571 {
                tunnel: w574 -> [_ w580]
                frame False {
                }
                frame True {
                  n276 = local write "Currently on Row"(w580) -> ()
                }
              }
              n277 = And(x=w571, y=w572) -> (x .and. y?=w570:bool)
            }
          }
          frame #1 {
            n278 = local read "Currently on Row"() -> (w586:i32)
            n279 = Increment(x=w586) -> (x+1=w585:i32)
            n280 = Index Array(array=w584, index=w585) -> (element=w587:T6)
            n281 = Unbundle By Name(w587) -> ("Row Type Selector"=w583:T8)
            n282 = Equal?(x=Multi_run_mode."Turn Off Row Repeating" ("Row Type Selector"), y=w583) -> (x = y?=w581:bool)
            n283 = while {
              shift-right: [w597] -> _
              shift-left: _ -> [w596]
              tunnel: w588 -> [w593]
              tunnel: w586 -> [w597]
              tunnel: w581 -> [w590]
              stop <- TRUE stop-if-true
              n284 = Decrement(x=w593) -> (x-1=w598:i32)
              n285 = Equal?(x=w597, y=w598) -> (x = y?=w591:bool)
              n286 = Not Equal?(x=w597, y=w596) -> (x != y?=w595:bool)
              n287 = Or(x=w590, y=w591) -> (x .or. y?=w589:bool)
              n288 = And(x=w595, y=w589) -> (x .and. y?=w594:bool)
              n289 = case shown="True" w594 {
                tunnel: w593 -> [_ w599]
                frame False {
                }
                frame True {
                  n290 = Initialize Array(timestamp(0 s since 1904-01-01) ("seconds since 1Jan1904"), w599) -> (w601:timestamp[])
                  n291 = global write "Trav_pos_global.vi" "Row completion times"(w601) -> ()
                }
              }
            }
          }
        }
      }
      frame "Which row to execute next" {
        # "Rep?"
        # "Repeat\nRow"
        n292 = local read "Currently on Row"() -> (w602:i32)
        n293 = stacked-sequence {
          seq-local: [_ w641 _] -> [_ _ w677]
          seq-local: [_ w640 _] -> [_ _ w678]
          seq-local: [w611 _ _] -> [_ w639 _]
          seq-local: [_ w636 _] -> [_ _ w671]
          tunnel: [w616 _ _] -> w608
          tunnel: w607 -> [w616 w643 w685]
          tunnel: w606 -> [_ _ w683]
          tunnel: w605 -> [_ w638 w684]
          tunnel: [_ _ w680] -> w604
          tunnel: w603 -> [_ _ w679]
          tunnel: w602 -> [w613 w635 w670]
          frame #0 {
            n294 = Array Size(array=w616) -> (size(s)=w615:i32)
            n295 = Decrement(x=w615) -> (x-1=w614:i32)
            n296 = Increment(x=w613) -> (x+1=w612:i32)
            n297 = while {
              tunnel: w612 -> [w620]
              tunnel: w616 -> [w632] mode=indexing
              tunnel: Multi_run_mode."Turn Off Row Repeating" ("Row Type Selector") -> [w631]
              tunnel: w614 -> [w627]
              tunnel: [w622] -> w611
              i -> [w624]
              stop <- w630 continue-if-true
              n298 = Less?(x=w624, y=w620) -> (x < y?=w625:bool)
              n299 = Unbundle By Name(w632) -> ("Row Type Selector"=w629:T8)
              n300 = Less?(x=w624, y=w627) -> (x < y?=w626:bool)
              n301 = Equal?(x=w624, y=w620) -> (x = y?=w621:bool)
              n302 = Equal?(x=w631, y=w629) -> (x = y?=w623:bool)
              n303 = case shown="True" w623 {
                tunnel: [TRUE w634] -> w622
                tunnel: w621 -> [_ w634]
                frame False {
                }
                frame True {
                }
              }
              n304 = Not(x=w623) -> (.not. x?=w628:bool)
              n305 = Compound Arithmetic op=AND(w628, w625, w626) -> (w630:bool)
            }
            n306 = global write "Trav_pos_global.vi" "Currently on point"(0 ("Currently on point")) -> ()
            n307 = global write "Trav_pos_global.vi" "Paused During Row?"(FALSE ("Paused During Row?")) -> ()
            n308 = global write "Trav_pos_global.vi" "Repeat Rows?"(w611) -> ()
          }
          frame #1 {
            n309 = global read "Trav_pos_global.vi" "Row completion times"() -> (w642:timestamp[])
            n310 = global read "Extra_Commands_Global.vi" "Minutes Before Repeating Row"() -> (w637:string)
            n311 = case shown="\"Run VI\"" w638 {
              tunnel: [w644 w645] -> w636
              frame "Check VI only" {
                n312 = global read "Trav_pos_global.vi" "Simulation Time"() -> (w644:timestamp)
              }
              frame "Run VI" {
                n313 = Get Date/Time In Seconds() -> (seconds since 1Jan1904=w645:timestamp)
                n314 = global write "Trav_pos_global.vi" "Simulation Time"(w645) -> ()
              }
            }
            n315 = while {
              tunnel: w643 -> [w655] mode=indexing
              tunnel: w642 -> [w658]
              tunnel: w636 -> [w657]
              tunnel: [w648] -> w641
              tunnel: [w647] -> w640
              tunnel: w639 -> [w651]
              tunnel: w635 -> [w649]
              tunnel: w637 -> [w646]
              i -> [w647]
              stop <- w654 continue-if-true
              n316 = Unbundle By Name(w655) -> ("Extra Commands"=w659:string)
              n317 = call "Extra_Commands.vi"("String to Search"=w659, "Command"=w646) -> ("Numeric Value"=w656:dbl, "Command Found"=w652:bool)  [unwired: 1 in, 3 out]
              n318 = And(x=w651, y=w652) -> (x .and. y?=w650:bool)
              n319 = case shown="True" w650 {
                tunnel: w658 -> [_ w665]
                tunnel: w657 -> [_ w666]
                tunnel: w647 -> [_ w664]
                tunnel: w656 -> [_ w662]
                tunnel: [FALSE w661] -> w648
                frame False {
                }
                frame True {
                  n320 = Index Array(array=w665, index=w664) -> (element=w667:timestamp)
                  n321 = Subtract(x=w666, y=w667) -> (x-y=w668:dbl)
                  n322 = Divide(x=w668, y=60.0) -> (x/y=w663:dbl)
                  n323 = Greater?(x=w663, y=w662) -> (0:w661:bool)
                }
              }
              n324 = Less?(x=w647, y=w649) -> (x < y?=w653:bool)
              n325 = Compound Arithmetic op=AND(invert w648, w653) -> (w654:bool)
            }
          }
          frame #2 {
            n326 = Not Equal?(x=w670, y=w678) -> (x != y?=w676:bool)
            n327 = And(x=w677, y=w676) -> (x .and. y?=w675:bool)
            n328 = case shown="False" w675 {
              tunnel: w678 -> [_ w711]
              tunnel: w670 -> [w707 w713]
              tunnel: [w706 w712] -> w681
              tunnel: [w706 w711] -> w672
              tunnel: w683 -> [w709 _]
              tunnel: [w705 TRUE] -> w682
              frame False {
                n329 = Increment(x=w707) -> (x+1=w708:i32)
                n330 = Greater?(x=w709, y=w708) -> (0:w705:bool)
                n331 = Select(t=w708, s=w705, f=w707) -> (s? t:f=w706:i32)
              }
              frame True {
                n332 = Greater?(x=w713, y=w711) -> (0:w714:bool)
                n333 = Select(t=w713, s=w714, f=w711) -> (s? t:f=w712:i32)
              }
            }
            n334 = global read "Trav_pos_global.vi" "Row completion times"() -> (w674:timestamp[])
            n335 = case shown="True" w682 {
              tunnel: w672 -> [_ w693]
              tunnel: w685 -> [_ w699]
              tunnel: w684 -> [w687 w691]
              tunnel: w681 -> [_ w697]
              tunnel: [w686 w696] -> w680
              tunnel: w679 -> [_ w696]
              frame False {
                n336 = case shown="\"Run VI\"" w687 {
                  tunnel: [Multi_Run_Case."Show jumped positions" ("Multi Run Case") Multi_Run_Case."Shut down source etc" ("Multi Run Case")] -> w686
                  frame "Check VI only" {
                  }
                  frame "Run VI" {
                  }
                }
              }
              frame True {
                n337 = Index Array(array=w699, index=w693) -> (element=w695:T6)
                n338 = Bundle By Name(cluster=w695, "Row No"=w693) -> (w694:T6)
                n339 = global write "Trav_pos_global.vi" "Meas Setup Number"(0 ("Meas Setup Number")) -> ()
                n340 = Build Array(w697) -> (w698:i32[])
                n341 = case shown="\"Run VI\"" w691 {
                  tunnel: w691 -> [_ w703]
                  tunnel: w694 -> [w700 w702]
                  tunnel: [w700 w701] -> w690
                  frame "Check VI only" {
                  }
                  frame "Run VI" {
                    n342 = call "Log_Current_row_to_Execute.vi"("Simulate/Run"=w703, "Start of Multi Run Prog"=FALSE, "Traverse line in"=w702) -> ("Traverse line Out"=w701:T6)  [unwired: 2 in, 4 out]
                  }
                }
                n343 = property on="Table" class="Arr (strict)"("Index Values"=w698) -> ()  [unwired: 2 in, 2 out]
                n344 = global write "Trav_pos_global.vi" "Current Row"(w690) -> ()
                "Currently on Row" <- w697
              }
            }
            n345 = Replace Array Subset(array=w674, new element=w671, index=w672) -> (w673:timestamp[])
            n346 = global write "Trav_pos_global.vi" "Row completion times"(w673) -> ()
          }
        }
      }
      frame "Evaluate IF Statement" {
        n347 = global read "Trav_pos_global.vi" "Current Row"() -> (w719:T6)
        n348 = Unbundle By Name(w719) -> ("Extra Commands"=w722:string)
        n349 = global read "Extra_Commands_Global.vi" "If Command"() -> (w725:string)
        n350 = call "Extra_Commands.vi"("String to Search"=w722, "Command"=w725) -> ("String Value"=w724:string, "Command Found"=w716:bool)  [unwired: 1 in, 3 out]
        n351 = Equal?(x=w720, y=User_Specific_mode."Run VI" ("Simulate/Run")) -> (x = y?=w715:bool)
        n352 = And(x=w716, y=w715) -> (x .and. y?=w717:bool)
        n353 = case shown="True" w717 {
          tunnel: w724 -> [_ w735]
          tunnel: [w731 w734] -> w718
          frame False {
            w731 = TRUE  # Execute Row?
          }
          frame True {
            n354 = call "Get_array_values_fr_String.vi"("String Value"=w735) -> ("Numeric Array"=w733:dbl[], "String array"=w732:string[])
            n355 = Index Array(array=w732, index=0 ("Index")) -> (element=w736:string)
            n356 = case shown="\"Global Value Between\"" w736 {
              tunnel: w735 -> [w741 _ _ _]
              tunnel: [w740 w742 w752 TRUE ("Execute Row?")] -> w734
              tunnel: w733 -> [_ w748 w766 _]
              tunnel: w732 -> [_ _ w760 _]
              frame "Time Between" {
                n357 = Get Date/Time In Seconds() -> (seconds since 1Jan1904=w738:timestamp)
                n358 = To Double Precision Float(number=w738) -> (double precision float=w739:dbl)
                n359 = call "If_Time_arguments.vi"("seconds since 1Jan1904"=w739, "String Value"=w741) -> ("Execute Row?"=w740:bool)  [unwired: 2 out]
              }
              frame "Global Value Between" {
                n360 = global read "Extra_Commands_Global.vi" "If command global value"() -> (w743:dbl)
                n361 = Index Array(array=w748, index=1 ("Index")) -> (element=w746:dbl)
                n362 = Index Array(array=w748, index=2 ("Index")) -> (element=w747:dbl)
                n363 = Max & Min(x=w746, y=w747) -> (max(x,y)=w745:dbl, min(x,y)=w744:dbl)
                n364 = In Range and Coerce(upper limit=w745, x=w743, lower limit=w744) -> (In Range?=w742:bool)  [unwired: 1 out]
              }
              frame "ADAM Channel Between" {
                n365 = Index Array(array=w760, index=1 ("Index")) -> (element=w759:string)
                n366 = Build Array(w759) -> (w758:string[])
                n367 = Index Array(array=w766, index=2 ("Index")) -> (element=w764:dbl)
                n368 = Index Array(array=w766, index=3 ("Index")) -> (element=w765:dbl)
                n369 = Max & Min(x=w764, y=w765) -> (max(x,y)=w763:dbl, min(x,y)=w762:dbl)
                n370 = call "Get_Current_Scan_client.vi"("ADAM Ch Names"=w758) -> ("Numerical Values"=w756:dbl[])  [unwired: 3 out]
                n371 = Index Array(array=w756, index=0 ("Index")) -> (element=w755:dbl)
                n372 = In Range and Coerce(upper limit=w763, x=w755, lower limit=w762) -> (In Range?=w753:bool)  [unwired: 1 out]
                n373 = Not A Number/Path/Refnum?(number/path/refnum=w755) -> (NaN/Path/Refnum?=w754:bool)
                n374 = Select(t=TRUE, s=w754, f=w753) -> (s? t:f=w752:bool)
              }
              frame "No Match", Default {
              }
            }
          }
        }
        n375 = Select(t=w728, s=w718, f=Multi_Run_Case."Calculate Row TIme" ("Multi Run Case")) -> (s? t:f=w727:T3)
      }
      frame "Perform Measurement Setup" {
        n376 = global read "Trav_pos_global.vi" "Current Row"() -> (w772:T6)
        n377 = case shown="\"Run VI\"" w771 {
          tunnel: w772 -> [_ w777]
          tunnel: w771 -> [_ w776]
          frame "Check VI only" {
          }
          frame "Run VI" {
            n378 = stacked-sequence {
              tunnel: w777 -> [w780 _]
              tunnel: w776 -> [w778 _]
              frame #0 {
                n379 = Unbundle By Name(w780) -> ("Extra Commands"=w779:string)
                n380 = call "Pause_for_server_ch_val.vi"("Extra command string"=w779, "Simulate/Run"=w778) -> ()  [unwired: 2 out]
              }
              frame #1 {
                n381 = Get Date/Time In Seconds() -> (seconds since 1Jan1904=w781:timestamp)
                n382 = To Double Precision Float(number=w781) -> (double precision float=w782:dbl)
                n383 = global write "Trav_pos_global.vi" "Start of Row time (Sec)"(w782) -> ()
              }
            }
          }
        }
      }
      frame "Set Measurement Conditions" {
        w788 = TRUE  # Row Completed
        w787 = FALSE  # Row Completed
        n384 = global read "Trav_pos_global.vi" "Current Row"() -> (w785:T6)
        n385 = Unbundle By Name(w785) -> ("Row Type Selector"=w790:T8)
        n386 = case shown="\"Run VI Named:\"" w790 {
          tunnel: [TRUE FALSE TRUE TRUE TRUE TRUE FALSE TRUE FALSE w839 FALSE FALSE FALSE] -> w795
          tunnel: w785 -> [w803 w806 w809 w812 w815 w818 w821 w824 w833 w838 w861 w864 w867]
          tunnel: [w803 w806 w809 w812 w815 w818 w821 w824 w832 w837 w861 w864 w867] -> w791
          tunnel: [w802 w805 w808 w811 w814 w817 w820 w823 w828 w835 w860 w863 w866] -> w789
          tunnel: w788 -> [w802 _ w808 w811 w814 _ _ _ _ w835 w860 w863 w866]
          tunnel: w787 -> [_ w805 _ _ _ w817 w820 w823 w828 _ _ _ _]
          tunnel: w784 -> [_ _ _ _ _ _ _ _ _ w836 _ _ _]
          frame "Move Traverse Only" {
          }
          frame "Check Beam Power" {
          }
          frame "Set Tunnel Speed Only" {
          }
          frame "Set Source Only" {
          }
          frame "Set Measurement Conditions" {
          }
          frame "Single Measurement" {
          }
          frame "Vertical Profile", Default {
          }
          frame "Scanning Valve Measurement" {
          }
          frame "Run VI Named:" {
            n387 = global read "Extra_Commands_Global.vi" "Skip Source Demand"() -> (w831:string)
            n388 = global read "Extra_Commands_Global.vi" "Establish Exp Conditions (s)"() -> (w827:string)
            n389 = Unbundle By Name(w833) -> ("Extra Commands"=w830:string)
            n390 = Concatenate Strings(w827, " = 0" ("Substring"), w831, w830) -> (w829:string)
            n391 = Bundle By Name(cluster=w833, "Extra Commands"=w829) -> (w832:T6)
          }
          frame "Send Message" {
            n392 = stacked-sequence {
              seq-local: [w840 _ _ _] -> [_ w845 _ _]
              tunnel: [_ _ _ FALSE] -> w839
              tunnel: w838 -> [_ w848 w854 w857]
              tunnel: [_ _ _ w857] -> w837
              tunnel: w836 -> [w841 _ _ _]
              frame #0 {
                n393 = Equal?(x=User_Specific_mode."Run VI" ("Simulate/Run"), y=w841) -> (x = y?=w840:bool)
              }
              frame #1 {
                n394 = Unbundle By Name(w848) -> ("Specific Arguments"=w846:string, "Filename"=w844:path)
                n395 = Build Array(w844) -> (w843:path[])
                n396 = case shown="True" w845 {
                  tunnel: "Message" ("Error Type") -> [_ w851]
                  tunnel: w846 -> [_ w850]
                  tunnel: w843 -> [_ w849]
                  frame False {
                  }
                  frame True {
                    n397 = call "Email_Text_Files.vi"("Filenames"=w849, "message"=w850, "subject ([No Subject])"=w851) -> ()
                  }
                }
              }
              frame #2 {
                n398 = global read "Extra_Commands_Global.vi" "Establish Exp Conditions (s)"() -> (w856:string)
                n399 = Unbundle By Name(w854) -> ("Extra Commands"=w855:string)
                n400 = call "Extra_Commands.vi"("String to Search"=w855, "Command"=w856) -> ("Numeric Value"=w852:dbl)  [unwired: 1 in, 4 out]
                n401 = call "Wait_Seconds_with_display.vi"("Message"="In Send Message Row", "Seconds to wait"=w852) -> ()  [unwired: 2 out]
              }
              frame #3 {
              }
            }
          }
          frame "Fall Back to this Row" {
          }
          frame "Turn Off Row Repeating" {
          }
          frame "Blank Row" {
          }
        }
        n402 = case shown="True" w795 {
          tunnel: w791 -> [_ w869]
          tunnel: w784 -> [_ w873]
          tunnel: [Multi_Run_Status."Continue" ("Status") w870] -> w783
          frame False {
          }
          frame True {
            w872 = 1  # Currently on Point
            n403 = call "Program_Active.vi"() -> ()  [unwired: 1 in]
            n404 = call "Set_Measurement_Conditions.vi"("Simulate/Run"=w873, "Currently on Point"=w872, "Traverse line"=w869) -> ("Status Cluster"=w871:T21)  [unwired: 2 out]
            n405 = Unbundle By Name(w871) -> ("Status"=w870:T2)
          }
        }
        n406 = case shown="\"Continue\"" w783 {
          tunnel: [w799 Multi_Run_Case."Calculate Row TIme" ("Multi Run Case")] -> w794
          tunnel: w793 -> [w800 _]
          tunnel: w789 -> [w797 _]
          frame "Continue" {
            n407 = Select(t=Multi_Run_Case."Calculate Row TIme" ("Multi Run Case"), s=w797, f=w800) -> (s? t:f=w799:T3)
          }
          frame "Jump to Next Point", Default {
          }
        }
        n408 = local write "Status"(w783) -> ()
      }
      frame "Execute Row" {
        n409 = global read "Trav_pos_global.vi" "Current Row"() -> (w875:T6)
        n410 = stacked-sequence {
          tunnel: w876 -> [w880 w891 w893]
          tunnel: w875 -> [w881 w888 w892]
          frame #0 {
            n411 = case shown="\"Check VI only\"" w880 {
              tunnel: w881 -> [w884 _]
              tunnel: w880 -> [w883 _]
              frame "Check VI only" {
                n412 = Unbundle By Name(w884) -> ("Extra Commands"=w885:string, "Row No"=w887:i32, "Meas Setup File"=w882:string)
                n413 = call "Skip_If Sd_Error_Below.vi"("String to Search"=w885, "Simulate/Run"=w883, "Measurement setup Applied?"=TRUE, "Row Number"=w887, "Measurement Setup File"=w882) -> ()  [unwired: 5 out]
              }
              frame "Run VI" {
              }
            }
          }
          frame #1 {
            n414 = call "Execute_Row.vi"("Simulate/Run"=w891, "Traverse line"=w888) -> ("Status"=w890:T2, "Traverse line out"=w889:T6)  [unwired: 2 out]
            n415 = global write "Trav_pos_global.vi" "Current Row"(w889) -> ()
            n416 = local write "Status"(w890) -> ()
          }
          frame #2 {
            w896 = FALSE  # Empty list
            n417 = call "Remember_RD_Folders.vi"("Empty list"=w896) -> ("List of Folders"=w895:path[])  [unwired: 1 in]
            n418 = for {
              tunnel: w892 -> [w901]
              tunnel: w895 -> [w900] mode=indexing
              tunnel: "Muti_Run_Log.xls" ("name or relative path") -> [w898]
              tunnel: w893 -> [w897]
              n419 = Build Path(base path=w900, name or relative path=w898) -> (appended path=w899:path)
              n420 = call "Log_Current_row_to_Execute.vi"("Simulate/Run"=w897, "Start of Multi Run Prog"=FALSE, "Traverse line in"=w901, "Multi Run Log File"=w899) -> ()  [unwired: 1 in, 5 out]
            }
          }
        }
      }
      frame "Calculate Row TIme" {
        n421 = global read "Trav_pos_global.vi" "Paused During Row?"() -> (w906:bool)
        n422 = local read "Status"() -> (w909:T2)
        n423 = global read "Trav_pos_global.vi" "Current Row"() -> (w905:T6)
        n424 = Equal?(x=w909, y=Multi_Run_Status."Continue" ("Status")) -> (x = y?=w908:bool)
        n425 = Equal?(x=w911, y=User_Specific_mode."Run VI" ("Simulate/Run")) -> (x = y?=w907:bool)
        n426 = Compound Arithmetic op=AND(w908, w907, invert w906) -> (w904:bool)
        n427 = case shown="False" w904 {
          tunnel: w905 -> [w924 w935]
          frame False {
            n428 = global read "Trav_pos_global.vi" "Simulation Time"() -> (w925:timestamp)
            n429 = To Double Precision Float(number=w925) -> (double precision float=w919:dbl)
            n430 = call "Calculate_Row_Time.vi"("Row Start Time (Sec Since 1904)"=w919, "Multi Run Row"=w924) -> ("Scalable Time (Sec)"=w922:dbl, "Fixed Time (Sec)"=w920:dbl)
            n431 = call "Overhead_Factor.vi"("Mode"=Overhead."Read Current Overhead") -> ("Current Overhead Factor"=w923:dbl)  [unwired: 3 in]
            n432 = Multiply(x=w923, y=w922) -> (x*y=w921:dbl)
            n433 = Add(x=w920, y=w921) -> (x+y=w916:dbl)
            n434 = global write "Trav_pos_global.vi" "Start of Row time (Sec)"(w916) -> ()
            n435 = Add(x=w919, y=w916) -> (x+y=w918:dbl)
            n436 = To Time Stamp(1:w918) -> (0:w917:timestamp)
            n437 = global write "Trav_pos_global.vi" "Simulation Time"(w917) -> ()
          }
          frame True {
            n438 = global read "Trav_pos_global.vi" "Start of Row time (Sec)"() -> (w933:dbl)
            n439 = Get Date/Time In Seconds() -> (seconds since 1Jan1904=w928:timestamp)
            n440 = To Double Precision Float(number=w928) -> (double precision float=w927:dbl)
            n441 = call "Calculate_Row_Time.vi"("Row Start Time (Sec Since 1904)"=w933, "Multi Run Row"=w935) -> ("Scalable Time (Sec)"=w929:dbl, "Fixed Time (Sec)"=w931:dbl)
            n442 = Subtract(x=w927, y=w933) -> (x-y=w932:dbl)
            n443 = Subtract(x=w932, y=w931) -> (x-y=w930:dbl)
            n444 = call "Overhead_Factor.vi"("Sum of Ideal times (Sec)"=w929, "Sum of Actual times (Sec)"=w930, "Mode"=Overhead."Update total times") -> ()  [unwired: 1 in, 1 out]
          }
        }
      }
      frame "Update time estimate" {
        n445 = global read "Trav_pos_global.vi" "Current Row"() -> (w939:T6)
        n446 = Unbundle By Name(w939) -> ("Row No"=w937:i32)
        n447 = local read "Currently on Row"() -> (w938:i32)
        n448 = Equal?(x=w937, y=w938) -> (x = y?=w936:bool)
        n449 = case shown="\"Run VI\"" w942 {
          tunnel: w945 -> [w953 w974]
          tunnel: [w952 w970] -> w944
          tunnel: w941 -> [_ w976]
          tunnel: [w951 w975] -> w940
          tunnel: w938 -> [w949 w969]
          tunnel: w939 -> [w950 w973]
          tunnel: w936 -> [w948 w972]
          frame "Check VI only" {
            n450 = global read "Trav_pos_global.vi" "Simulation Time"() -> (w955:timestamp)
            n451 = To Double Precision Float(number=w955) -> (double precision float=w954:dbl)
            n452 = call "Sec_to_date_filename.vi"("seconds"=w954) -> ("Day"=w957:string, "Time"=w956:string)  [unwired: 2 out]
            n453 = Concatenate Strings(w956, "  " ("Substring"), w957) -> (w951:string)
            n454 = case shown="True" w948 {
              tunnel: w949 -> [_ w968]
              tunnel: w953 -> [w959 w967]
              tunnel: [w959 w965] -> w952
              tunnel: w951 -> [_ w964]
              tunnel: w950 -> [_ w963]
              frame False {
              }
              frame True {
                n455 = global read "Trav_pos_global.vi" "Start of Row time (Sec)"() -> (w962:dbl)
                n456 = Divide(x=w962, y=60.0) -> (x/y=w960:dbl)
                n457 = Bundle By Name(cluster=w963, "Completion time"=w964, "Row Duration (mins)"=w960) -> (w966:T6)
                n458 = Replace Array Subset(array=w967, new element=w966, index=w968) -> (w965:T6[])
              }
            }
          }
          frame "Run VI" {
            n459 = case shown="True" w972 {
              tunnel: w969 -> [_ w983]
              tunnel: w974 -> [w979 w982]
              tunnel: w973 -> [_ w981]
              tunnel: [w979 w980] -> w971
              frame False {
              }
              frame True {
                n460 = Replace Array Subset(array=w982, new element=w981, index=w983) -> (w980:T6[])
              }
            }
            n461 = call "Calc_Remaining_Time.vi"("Currently on Row"=w969, "Table In"=w971) -> ("Table Out"=w970:T6[])  [unwired: 1 out]
            n462 = Decrement(x=w976) -> (x-1=w978:i32)
            n463 = Index Array(array=w970, index=w978) -> (element=w977:T6)
            n464 = Unbundle By Name(w977) -> ("Completion time"=w975:string)
          }
        }
        "Estimated Completion time" <- w940
        n465 = global write "Trav_pos_global.vi" "Estimated Completion time"(w940) -> ()
      }
      frame "Pause Multi Run Program" {
        n466 = while {
          tunnel: "Pause" -> [w995]
          tunnel: [w998] -> w990
          tunnel: w989 -> [w997]
          tunnel: w987 -> [w996]
          shift-right: [w995] -> _
          shift-left: _ -> [w994]
          stop <- TRUE stop-if-true
          n467 = case shown="True" w995 {
            tunnel: [w999 w1004] -> w998
            tunnel: w997 -> [w999 w1002]
            tunnel: w996 -> [_ w1003]
            tunnel: w995 -> [_ w1001]
            tunnel: w994 -> [_ w1000]
            frame False {
            }
            frame True {
              n468 = stacked-sequence {
                tunnel: w1002 -> [_ _ _ _ w1019]
                tunnel: [_ _ _ _ w1020] -> w1004
                tunnel: w1003 -> [w1006 _ _ _ _]
                tunnel: w1001 -> [_ _ _ w1015 _]
                tunnel: w1000 -> [_ _ _ w1014 _]
                frame #0 {
                  n469 = Quotient & Remainder(x=w1006, y=15) -> (x-y*floor(x/y)=w1005:i32)  [unwired: 1 out]
                  n470 = case shown="0" w1005 {
                    frame 0 {
                      n471 = Current VI's Path() -> (path=w1008:path)
                      n472 = call "Bring_to_front.vi"("path"=w1008) -> ()
                    }
                    frame 1, Default {
                    }
                  }
                }
                frame #1 {
                  n473 = global write "Trav_pos_global.vi" "Paused During Row?"(TRUE ("Paused During Row?")) -> ()
                  "Pause message" <- "Multi Run Program Paused!!!!" ("Pause message")
                }
                frame #2 {
                  n474 = property on="Pause message" class="Str"("Visible"=TRUE) -> ()  [unwired: 2 in, 2 out]
                  n475 = Wait Until Next ms Multiple(millisecond multiple=u32 1500) -> ()  [unwired: 1 out]
                }
                frame #3 {
                  n476 = Compound Arithmetic op=AND(w1015, invert w1014) -> (w1013:bool)
                  n477 = case shown="True" w1013 {
                    frame False {
                    }
                    frame True {
                      n478 = call "Program_Active_Client.vi"("Mode"=enum16{"Program Active", "Traverse Level State"}."Program Active", "Time till next contact (Sec)"=12000.0, "Traverse level State"=Traverse_Level_State."Running") -> ()  [unwired: 3 out]
                    }
                  }
                }
                frame #4 {
                  n479 = property on="Pause message" class="Str"("Visible"=FALSE) -> ()  [unwired: 2 in, 2 out]
                  n480 = Wait Until Next ms Multiple(millisecond multiple=u32 1500) -> ()  [unwired: 1 out]
                  n481 = Decrement(x=w1019) -> (x-1=w1020:T3)
                }
              }
            }
          }
        }
        n482 = call "Overhead_Factor.vi"("Mode"=Overhead."Read Current Overhead") -> ("Current Overhead Factor"=→"Current Overhead Factor":dbl)  [unwired: 3 in]
      }
      frame "Do Another Row?" {
        w1033 = Multi_Run_Status."Terminate Run" ("Status")
        n483 = case shown="False" "Stop after Repeats" {
          tunnel: [w1041 w1042] -> w1027
          tunnel: w1023 -> [_ w1043]
          frame False {
            n484 = local read "Currently on Row"() -> (w1041:i32)
            n485 = Increment(x=w1041) -> (x+1=→"Last Row Run":i32)
          }
          frame True {
            n486 = Decrement(x=w1043) -> (x-1=w1042:i32)
            n487 = local write "Currently on Row"(w1042) -> ()
          }
        }
        n488 = case shown="False" "stop" {
          tunnel: [w1044 w1045] -> w1034
          tunnel: w1033 -> [_ w1045]
          frame False {
            n489 = local read "Status"() -> (w1044:T2)
          }
          frame True {
            n490 = local write "Status"(w1045) -> ()
          }
        }
        n491 = Not Equal?(x=w1034, y=w1033) -> (x != y?=w1032:bool)
        n492 = Increment(x=w1027) -> (x+1=w1026:i32)
        n493 = Index Array(array=w1028, index=w1026) -> (element=w1025:T6)
        n494 = Unbundle By Name(w1025) -> ("Row Type Selector"=w1031:T8)
        n495 = Equal?(x=w1031, y=Multi_run_mode."Turn Off Row Repeating" ("Row Type Selector")) -> (x = y?=w1029:bool)
        n496 = case shown="True" w1032 {
          tunnel: [w1046 w1050] -> w1038
          tunnel: w1027 -> [_ _]
          tunnel: w1037 -> [w1047 _]
          tunnel: w1028 -> [_ _]
          tunnel: w1034 -> [_ w1051]
          tunnel: w1023 -> [_ _]
          tunnel: w1029 -> [_ _]
          frame False {
            n497 = case shown="\"Check VI only\"" w1047 {
              tunnel: [Multi_Run_Case."Show jumped positions" ("Multi Run Case") Multi_Run_Case."Shut down source etc" ("Multi Run Case")] -> w1046
              frame "Check VI only" {
              }
              frame "Run VI" {
              }
            }
          }
          frame True {
            n498 = case shown="\"Jump To Fall Back\"" w1051 {
              tunnel: [Multi_Run_Case."Skip Blank Rows" ("Multi Run Case") Multi_Run_Case."Find Next Fall Back Row" ("Multi Run Case")] -> w1050
              frame "Continue", Default {
              }
              frame "Jump To Fall Back" {
              }
            }
          }
        }
      }
      frame "Find Next Fall Back Row" {
        n499 = local read "Currently on Row"() -> (w1055:i32)
        n500 = Increment(x=w1055) -> (x+1=w1054:i32)
        n501 = Index Array(array=w1063, index=w1055) -> (element=w1064:T6)
        n502 = Array Size(array=w1063) -> (size(s)=w1062:i32)
        n503 = Unbundle By Name(w1064) -> ("Row Type Selector"=w1058:T8)
        n504 = Greater?(x=w1062, y=w1054) -> (0:w1061:bool)
        n505 = Equal?(x=w1058, y=Multi_run_mode."Fall Back to this Row" ("Mode")) -> (x = y?=w1056:bool)
        n506 = case shown="True" w1061 {
          tunnel: [Multi_Run_Case."Skip Blank Rows" ("Multi Run Case") w1071] -> w1060
          tunnel: w1056 -> [_ w1067]
          tunnel: w1055 -> [_ w1068]
          frame False {
          }
          frame True {
            n507 = case shown="False" w1067 {
              tunnel: w1068 -> [w1073 _]
              frame False {
                n508 = Increment(x=w1073) -> (x+1=w1072:i32)
                n509 = local write "Currently on Row"(w1072) -> ()
              }
              frame True {
              }
            }
            n510 = Select(t=Multi_Run_Case."Skip Blank Rows" ("Multi Run Case"), s=w1067, f=Multi_Run_Case."Find Next Fall Back Row" ("Multi Run Case")) -> (s? t:f=w1071:T3)
          }
        }
      }
      frame "Shut down source etc" {
        n511 = for {
          tunnel: w1093 -> [w1112] mode=indexing
          tunnel: Multi_run_mode."Synchronize With:" ("Mode") -> [w1110]
          tunnel: [w1109] -> w1095 mode=indexing
          n512 = Unbundle By Name(w1112) -> ("Row Type Selector"=w1111:T8)
          n513 = Equal?(x=w1111, y=w1110) -> (x = y?=w1109:bool)
        }
        n514 = call "Overhead_Factor.vi"("Mode"=Overhead."Re Scale totals to 3 hrs") -> ()  [unwired: 3 in, 1 out]
        n515 = local read "Status"() -> (w1081:T2)
        n516 = call "Set_Source.vi"("Source Status"=Client_Source_Status."Not Using", "Simulate/Run"=w1084) -> ("Status Cluster"=w1085:T21)  [unwired: 2 in, 5 out]
        n517 = call "Program_Active_Client.vi"("Mode"=enum16{"Program Active", "Traverse Level State"}."Traverse Level State", "Traverse level State"=Traverse_Level_State."Complete") -> ()  [unwired: 1 in, 3 out]
        n518 = global read "Meas_global.vi" "Start Time of experiment"() -> (w1091:dbl)
        n519 = Equal?(x=w1081, y=Multi_Run_Status."Terminate Run" ("Status")) -> (x = y?=w1079:bool)
        n520 = call "Prog_Status_Handler.vi"("Status Cluster"=w1085, "Simulate/Run"=w1084) -> ()  [unwired: 2 out]
        n521 = global read "Meas_global.vi" "LDA data"() -> (w1100:enum16{"No LDA data", "Take LDA data"})
        n522 = Or Array Elements(Boolean array=w1095) -> (logical OR=w1082:bool)
        n523 = Get Date/Time In Seconds() -> (seconds since 1Jan1904=w1074:timestamp)
        n524 = Compound Arithmetic op=AND(w1082, invert w1079) -> (w1083:bool)
        n525 = To Double Precision Float(number=w1074) -> (double precision float=w1092:dbl)
        n526 = case shown="\"Take LDA data\"" w1100 {
          frame "No LDA data" {
          }
          frame "Take LDA data" {
            w1113 = FALSE  # High Voltage
            w1118 = 0.0  # Input
            n527 = global read "LDA_meas_global_2.vi" "BSA2 info"() -> (w1115:T22)
            n528 = global read "LDA_meas_global_1.vi" "BSA1 info"() -> (w1117:T22)
            n529 = Unbundle By Name(w1115) -> ("GPIB Address"=w1114:string)
            n530 = Unbundle By Name(w1117) -> ("GPIB Address"=w1116:string)
            n531 = call "Hydrosonic_Conrol.vi"("Input Mode"=enum16{"Desired Frequency", "Transducer value"}."Transducer value", "Desired Value"=w1118) -> ()  [unwired: 2 in, 2 out]
            n532 = call "Set_BSA_voltage_On_Off.vi"("GPIB address"=w1116, "High Voltage"=w1113) -> ()  [unwired: 1 in, 5 out]
            n533 = call "Set_BSA_voltage_On_Off.vi"("GPIB address"=w1114, "High Voltage"=w1113) -> ()  [unwired: 1 in, 5 out]
          }
        }
        n534 = case shown="True" w1083 {
          frame False {
          }
          frame True {
            n535 = global read "Preference_global.vi" "Rig Setup"() -> (w1102:string)
            n536 = Concatenate Strings(w1102, ":Program:Sync") -> (w1104:string)
            n537 = Bundle By Name(cluster=T19 {"Channel Name"="", "New Value"=0.0} ("Update Scan Value Cluster"), "Channel Name"=w1104, "New Value"=1000.0 ("Bundle Element")) -> (w1105:T19)
            n538 = Build Array(w1105) -> (w1107:T19[])
            n539 = call "Update_Current_Value_client.vi"("Update array in"=w1107) -> ()  [unwired: 1 in]
          }
        }
        n540 = Subtract(x=w1092, y=w1091) -> (x-y=w1090:dbl)
        n541 = Greater?(x=w1090, y=300.0) -> (0:w1087:bool)
        n542 = Not(x=w1087) -> (.not. x?=→"Non Starter":bool)
        n543 = Increment(x=w1077) -> (x+1=w1076:T3)
        n544 = Increment(x=w1076) -> (x+1=w1075:T3)
        n545 = Select(t=w1077, s=w1087, f=w1075) -> (s? t:f=w1088:T3)
      }
      frame "Email results to users" {
        n546 = local read "Currently on Row"() -> (w1125:i32)
        n547 = Increment(x=w1125) -> (x+1=w1120:i32)
        n548 = Split 1D Array(array=w1122, index=w1120) -> (first subarray=w1129:T6[], second subarray=w1128:T6[])
        n549 = Array Size(array=w1128) -> (size(s)=w1130:i32)
        n550 = for {
          tunnel: w1129 -> [w1145] mode=indexing
          shift-right: [w1143] -> w1131
          shift-left: string[] [] -> [w1144]
          n551 = Unbundle By Name(w1145) -> ("Row Type Selector"=w1136:T8, "Filename"=w1142:path, "Comments"=w1141:string)
          n552 = Not Equal?(x=Multi_run_mode."Auto Calibrate" ("Row Type Selector"), y=w1136) -> (x != y?=w1138:bool)
          n553 = Empty String/Path?(string/path=w1142) -> (empty?=w1139:bool)
          n554 = Compound Arithmetic op=AND(w1138, invert w1139) -> (w1137:bool)
          n555 = case shown="True" w1137 {
            tunnel: w1144 -> [w1146 w1154]
            tunnel: [w1146 w1153] -> w1143
            tunnel: w1142 -> [_ w1152]
            tunnel: w1141 -> [_ w1150]
            frame False {
            }
            frame True {
              n556 = Path To String(path=w1152) -> (string=w1151:string)
              n557 = Match Pattern(string=w1150, regular expression=" !!Program added comments") -> (after substring=w1147:string)  [unwired: 4 out]
              n558 = Concatenate Strings(w1151, w1147) -> (w1149:string)
              n559 = Build Array (concatenate)(w1154, w1149) -> (w1153:string[])
            }
          }
        }
        n560 = Equal To 0?(x=w1130) -> (x = 0?=w1121:bool)
        n561 = case shown="False" w1121 {
          tunnel: ["Having completed only some of the requested rows." ("Message") ""] -> w1126
          frame False {
          }
          frame True {
          }
        }
        n562 = call "End_of_run_messages.vi"("Message"=w1126, "Subject"="Multi Run Ended", "Attachments"=w1131) -> ()  [unwired: 1 in]
      }
      frame "Save run efficiency" {
        w1166 = FALSE  # append to file? (new file:F)
        w1165 = FALSE  # advisory dialog? (display:T)
        n563 = call "Setup_Filepath.vi"("Setup File Type"=Setup_Filetype."General", "Filename in"="Preferences.xls" ("name or relative path")) -> ("Filename Out"=w1155:path)  [unwired: 1 out]
        n564 = call "Overhead_Factor.vi"("Mode"=Overhead."Read Current Overhead") -> ("Current Overhead Factor"=w1160:dbl)  [unwired: 3 in]
        n565 = Number To Fractional String(number=w1160, precision (6)=i16 4) -> (F-format string=w1158:string)  [unwired: 2 out]
        n566 = call "Read_Characters_From_File.ph.vi"("file path (dialog if empty)"=w1155) -> ("character string"=w1163:string)  [unwired: 1 in, 7 out]
        n567 = call "Replace_data_in_setup_string.vi"("New data string"=w1158, "Input string"=w1163, "Variable name"="Current Overhead Factor") -> ("Appended string"=w1162:string)
        n568 = call "Write_Characters_To_File.vi"("file path (dialog if empty)"=w1155, "advisory dialog? (display:T)"=w1165, "character string"=w1162, "append to file? (new file:F)"=w1166) -> ()  [unwired: 1 in, 4 out]
      }
      frame "Remove Skipped Commands" {
        n569 = for {
          tunnel: w1172 -> [w1180] mode=indexing
          tunnel: [w1179] -> w1171 mode=indexing
          n570 = Unbundle By Name(w1180) -> ("Comments"=w1178:string)
          n571 = Match Pattern(string=w1178, regular expression=" !!Program added comments") -> (before substring=w1177:string)  [unwired: 4 out]
          n572 = Bundle By Name(cluster=w1180, "Comments"=w1177) -> (w1179:T6)
        }
      }
      frame "Show jumped positions" {
        n573 = global read "Trav_pos_global.vi" "Jumped Positions"() -> (w1183:dbl[][])
        n574 = Array Size(array=w1183) -> (size(s)=w1186:i32[])
        n575 = Index Array(array=w1186, index=0) -> (element=w1182:i32)
        n576 = Greater Than 0?(x=w1182) -> (x > 0?=w1184:bool)
        n577 = case shown="True" w1184 {
          tunnel: w1183 -> [_ w1197]
          tunnel: w1182 -> [_ w1196]
          frame False {
            w1190 = TRUE  # Front Panel Window:Is Frontmost
            n578 = Current VI's Path() -> (path=w1191:path)
            n579 = Open VI Reference(vi path=w1191) -> (vi reference=w1192:refnum<vi>, error out=w1193:errorcluster)  [unwired: 1 in, 4 out]
            n580 = property class="VI"(reference=w1192, error in=w1193, "Front Panel Window:Is Frontmost"=w1190) -> (reference out=w1194:refnum<vi>, error out=w1195:errorcluster)
            n581 = Close Reference(reference=w1194, error in (no error)=w1195) -> ()  [unwired: 1 out]
          }
          frame True {
            n582 = stacked-sequence {
              tunnel: w1197 -> [w1198 w1208]
              tunnel: w1196 -> [w1202 _]
              frame #0 {
                n583 = global read "Trav_pos_global.vi" "Default Traverse Setup"() -> (w1199:string)
                n584 = Format Into String(format string="There are %d points which cannot be reached", w1202) -> (resulting string=w1200:string)  [unwired: 2 in, 1 out]
                n585 = call "Display_Trav_Views.vi"("Current Probe Position"=w1198, "Traverse Name"=w1199, "Open Front Panel"=TRUE, "Error Comments"=w1200, "Crash?"=FALSE) -> ()  [unwired: 2 in, 4 out]
              }
              frame #1 {
                n586 = local read "Command filename"() -> (w1212:path)
                n587 = Array To Spreadsheet String(array=w1208, 3:"%.1f" ("format string")) -> (spreadsheet string=w1206:string)  [unwired: 1 out]
                n588 = Strip Path(path=w1212) -> (stripped path=w1211:path)  [unwired: 1 out]
                n589 = Build Path(base path=w1211, name or relative path="Jumped_Positions.xls") -> (appended path=w1209:path)
                n590 = call "Write_File_Simple.vi"("append to file? (new file:F)"=FALSE, "character string"=w1206, "file path"=w1209) -> ()  [unwired: 2 out]
              }
            }
          }
        }
      }
      frame "Save Setup to File" {
        w1229 = FALSE  # Start of Multi Run Prog
        n591 = Array Size(array=w1243) -> (size(s)=w1248:i32)
        n592 = local read "Last Row Run"() -> (w1218:i32)
        n593 = local read "Status"() -> (w1224:T2)
        n594 = local read "Stop after Repeats"() -> (w1227:bool)
        n595 = local read "stop"() -> (w1228:bool)
        n596 = Decrement(x=w1218) -> (x-1=w1219:i32)
        n597 = Increment(x=w1219) -> (x+1=w1231:i32)
        n598 = local read "Command filename"() -> (w1214:path)
        n599 = Equal?(x=w1224, y=Multi_Run_Status."Continue" ("Status")) -> (x = y?=w1223:bool)
        n600 = Compound Arithmetic op=OR(w1227, w1228, w1223) -> (w1226:bool)
        n601 = local read "Non Starter"() -> (w1236:bool)
        n602 = Select(t=w1231, s=w1226, f=w1219) -> (s? t:f=w1230:i32)
        n603 = Less?(x=w1222, y=T9."Run Multi Run Prog") -> (x < y?=w1220:bool)
        n604 = Equal?(x=w1248, y=w1218) -> (x = y?=w1238:bool)
        n605 = Equal To 0?(x=w1231) -> (x = 0?=w1237:bool)
        n606 = Split 1D Array(array=w1243, index=w1230) -> (second subarray=w1246:T6[])  [unwired: 1 out]
        n607 = Compound Arithmetic op=OR(w1238, w1237, w1236, w1220) -> (w1239:bool)
        n608 = call "Current_Filepath.vi"("Filename in"=w1214, "Data Type"="Commands") -> ("Filename Out"=w1213:path)  [unwired: 1 out]
        n609 = local read "Work in Tunnel Coordinates?"() -> (w1217:T1)
        n610 = local read "Jump Bad Positions"() -> (w1216:bool)
        n611 = case shown="False" w1239 {
          tunnel: w1213 -> [w1256 w1289]
          tunnel: [w1255 w1289] -> w1247
          tunnel: w1246 -> [w1253 _]
          tunnel: [w1252 w1290] -> w1245
          tunnel: w1243 -> [w1254 w1290]
          tunnel: w1217 -> [w1251 _]
          tunnel: w1216 -> [w1250 _]
          frame False {
            n612 = stacked-sequence {
              tunnel: w1256 -> [w1257 w1268 _]
              tunnel: [_ w1261 _] -> w1255
              tunnel: w1254 -> [w1260 _ w1273]
              tunnel: w1253 -> [_ _ w1271]
              tunnel: [_ _ w1270] -> w1252
              tunnel: w1251 -> [w1259 _ _]
              tunnel: w1250 -> [w1258 _ _]
              frame #0 {
                n613 = call "Save_Trav_setup.vi"("Work in Tunnel Coordinates?"=w1259, "Trav Table"=w1260, "Jump Bad Positions"=w1258, "Setup filename"=w1257) -> ()  [unwired: 2 out]
              }
              frame #1 {
                n614 = Strip Path(path=w1268) -> (stripped path=w1269:path, name=w1267:string)
                n615 = call "Add_filename_suffix.vi"("Filename"=w1267) -> ("Original Suffix"=w1264:string, "Base name"=w1266:string)  [unwired: 1 in, 2 out]
                n616 = Concatenate Strings(w1266, "_Rem", w1264) -> (w1263:string)
                n617 = Build Path(base path=w1269, name or relative path=w1263) -> (appended path=w1262:path)
                n618 = call "Find_Unique_Filename.vi"("Path In"=w1262) -> ("Unique Path Out"=w1261:path)  [unwired: 1 in, 1 out]
              }
              frame #2 {
                n619 = Index Array(array=w1273, index=0) -> (element=w1276:T6)
                n620 = Initialize Array(w1276, 0 ("dimension size")) -> (w1275:T6[])
                n621 = global read "Extra_Commands_Global.vi" "Minutes Before Repeating Row"() -> (w1274:string)
                n622 = for {
                  shift-right: [w1279] -> w1272
                  shift-left: w1275 -> [w1281]
                  tunnel: w1274 -> [w1283]
                  tunnel: w1273 -> [w1280] mode=indexing
                  n623 = Unbundle By Name(w1280) -> ("Extra Commands"=w1282:string)
                  n624 = call "Extra_Commands.vi"("String to Search"=w1282, "Command"=w1283) -> ("Command Found"=w1284:bool)  [unwired: 1 in, 4 out]
                  n625 = case shown="False" w1284 {
                    tunnel: w1281 -> [w1285 w1288]
                    tunnel: w1280 -> [_ w1287]
                    tunnel: [w1285 w1286] -> w1279
                    frame False {
                    }
                    frame True {
                      n626 = Build Array (concatenate)(w1288, w1287) -> (w1286:T6[])
                    }
                  }
                }
                n627 = Build Array (concatenate)(w1272, w1271) -> (w1270:T6[])
              }
            }
          }
          frame True {
          }
        }
        n628 = Path To String(path=w1213) -> (string=w1235:string)
        n629 = Concatenate Strings("Multi run Prog Ended having the setup filename of :" ("Message"), w1235) -> (w1234:string)
        n630 = call "Save_Trav_setup.vi"("Work in Tunnel Coordinates?"=w1217, "Trav Table"=w1245, "Jump Bad Positions"=w1216, "Setup filename"=w1247) -> ("Trav Table Out"=w1244:T6[])  [unwired: 1 out]
        n631 = call "Log_Current_row_to_Execute.vi"("Simulate/Run"=w1233, "Message"=w1234, "Start of Multi Run Prog"=w1229) -> ()  [unwired: 2 in, 5 out]
        n632 = Select(t=w1244, s=w1239, f=w1243) -> (s? t:f=w1242:T6[])
      }
      frame "End" {
        w1292 = ""
        w1294 = path ""
        w1295 = 0 ("No. of pts.")
        w1297 = nan
        n633 = global write "Trav_pos_global.vi" "Top level setup filename"(w1294) -> ()
        n634 = global read "Trav_pos_global.vi" "Current Row"() -> (w1301:T6)
        n635 = Bundle By Name(cluster=w1301, "Start X"=w1297, "Start Y"=w1297, "Start Z"=w1297, "End X"=w1297, "End Y"=w1297, "End Z"=w1297, "No. of pts."=w1295, "Spacing"=Spacing."Linear", "Filename"=w1294, "Tunnel Speed"=w1297, "Averaging time (min)"=w1297, "Extra Commands"=w1292, "Specific Arguments"=w1292, "Emission Rate (l/min)"=w1297, "Trace Gas Concentration (%)"=w1297, "Density Ratio"=w1292, "Comments"=w1292, "Row No"=w1295, "Row Type Selector"=Multi_run_mode."Blank Row", "Completion time"=w1292, "Meas Setup File"=w1292, "Row Duration (mins)"=w1297, "No. of Valid pts."=w1295) -> (w1300:T6)
        n636 = Current VI's Path() -> (path=w1293:path)
        n637 = global write "Trav_pos_global.vi" "Current Row"(w1300) -> ()
        n638 = global write "Trav_pos_global.vi" "Meas Setup Number"(0 ("Meas Setup Number")) -> ()
        n639 = call "Bring_to_front.vi"("path"=w1293) -> ()
        n640 = global write "Trav_pos_global.vi" "Estimated Completion time"("") -> ()
        n641 = Build Array(u32 0) -> (w1302:u32[])
        n642 = property on="Table" class="Arr (strict)"("Index Values"=w1302) -> ()  [unwired: 2 in, 2 out]
      }
    }
    n643 = case shown="False" w8 {
      tunnel: w4 -> [_ w15]
      frame False {
      }
      frame True {
        n644 = local write "Table"(w15) -> ()
      }
    }
    "Multi Run Case" <- w10
  }
